vi "WVDIAL_Main.vi"() -> ()   [LabVIEW 2024]
uses:
  TypeDefinitions.llb/TypeDef_MainControlSystem.ctl
  TypeDefinitions.llb/TypeDef_LoopStagesMain.ctl
  <vilib>/Utility/miscctls.llb/LVRectTypeDef.ctl
  <vilib>/Utility/miscctls.llb/LVPointTypeDef.ctl
  TypeDefinitions.llb/TypeDef_ConfigureFIleTypes.ctl
  TypeDefinitions.llb/TypeDef_ChildReporting.ctl
  TypeDefinitions.llb/TypeDef_MainSpecialConfiguration.ctl
  WVDIAL_GlobalVariables.vi
panel:
  out "ChildrenDetails":T2(array[cluster])
  in  "Software Testing":bool
  out "Pages":refnum<vi>[](array[refnum])
  out "SubPanelRefs":refnum<vi>[](array[refnum])
  out "SubPanelWidth":i32=985
  out "SubPanelHeight":i32=540
  out "error IO":errorcluster
  out "Children Responding":T3(array[cluster])
  out "QueueElement":string="Exit"
  out "LoopCounter":i32=200
  out "Permission Level":T4(ring)
  in  "User Comment":bool
  in  "Update Permissions":bool
  in  "Global Abort":bool=TRUE
  in  "Tab Control":T5(tab)
  in  "BDetector":bool=TRUE
  in  "DopFreeScan":bool=TRUE
  out "Doppler Free Calibration":bool
  out "Receiver Calibration":bool
  in  "AfterPulse Calibration":bool
  in  "Aerodiode":bool=TRUE
  in  "TCSPC":bool=TRUE
  in  "CurrentSensor":bool=TRUE
  in  "ConfigThor8000":bool=TRUE caption="ConfigQC"
  in  "ConfigQC":bool=TRUE
  in  "Switches":bool=TRUE
  in  "Wavemeter":bool=TRUE
  in  "Thor8000":bool=TRUE
  in  "PowerSwitches":bool=TRUE
  in  "SetupRScan":bool=TRUE
  in  "Housekeeping":bool=TRUE
  in  "Operations":bool=TRUE
  in  "Warmup":bool=TRUE
  out "DIAL unit":string="DIAL5"
  out "UPSAbort":bool
  in  "NetCDF":bool=TRUE
  in  "Thermocouples":bool=TRUE
  in  "LaserLocking":bool=TRUE
  in  "MCS":bool=TRUE
  in  "Weather Station":bool=TRUE
  in  "QComposer":bool=TRUE
  in  "UPS":bool=TRUE
  in  "Humidity":bool=TRUE
  in  "Template":bool=TRUE
  out "What to Do":string
  out "WritePaths":path[](array[path])=[path "C:/Users/h2odial/Desktop/WVDCode/WVD-MCSupdate/WVDNewArchitectureUpdate/WVD_Architecture_Update/Data/Container/20181008/ContainerLogging_20181008_155204.txt"]
  out "DataBasePath":string="C:\\Users\\h2odial\\Desktop\\WVDCode\\WVD-MCSupdate\\WVDNewArchitectureUpdate\\WVD_Architecture_Update\\Data\\Container\\"
  out "FileBaseNames":string[](array[string])=["ContainerLogging"]
  out "FileUpdateTime":dbl=15.867789441666668
  in  "TempScan":bool=TRUE
  out "First/LastCall":bool
  out "Configuration":enum16{"Ops", "ReceiverScan"}(ring)
  in  "PulsedScan":bool=TRUE
  # "Place Hidden Variables Here"
  # "Main Programs"
  # "Testing Programs"
  # "Hardware Setup Programs"
  # "Individual Controls"
  # "Calibration  Programs"
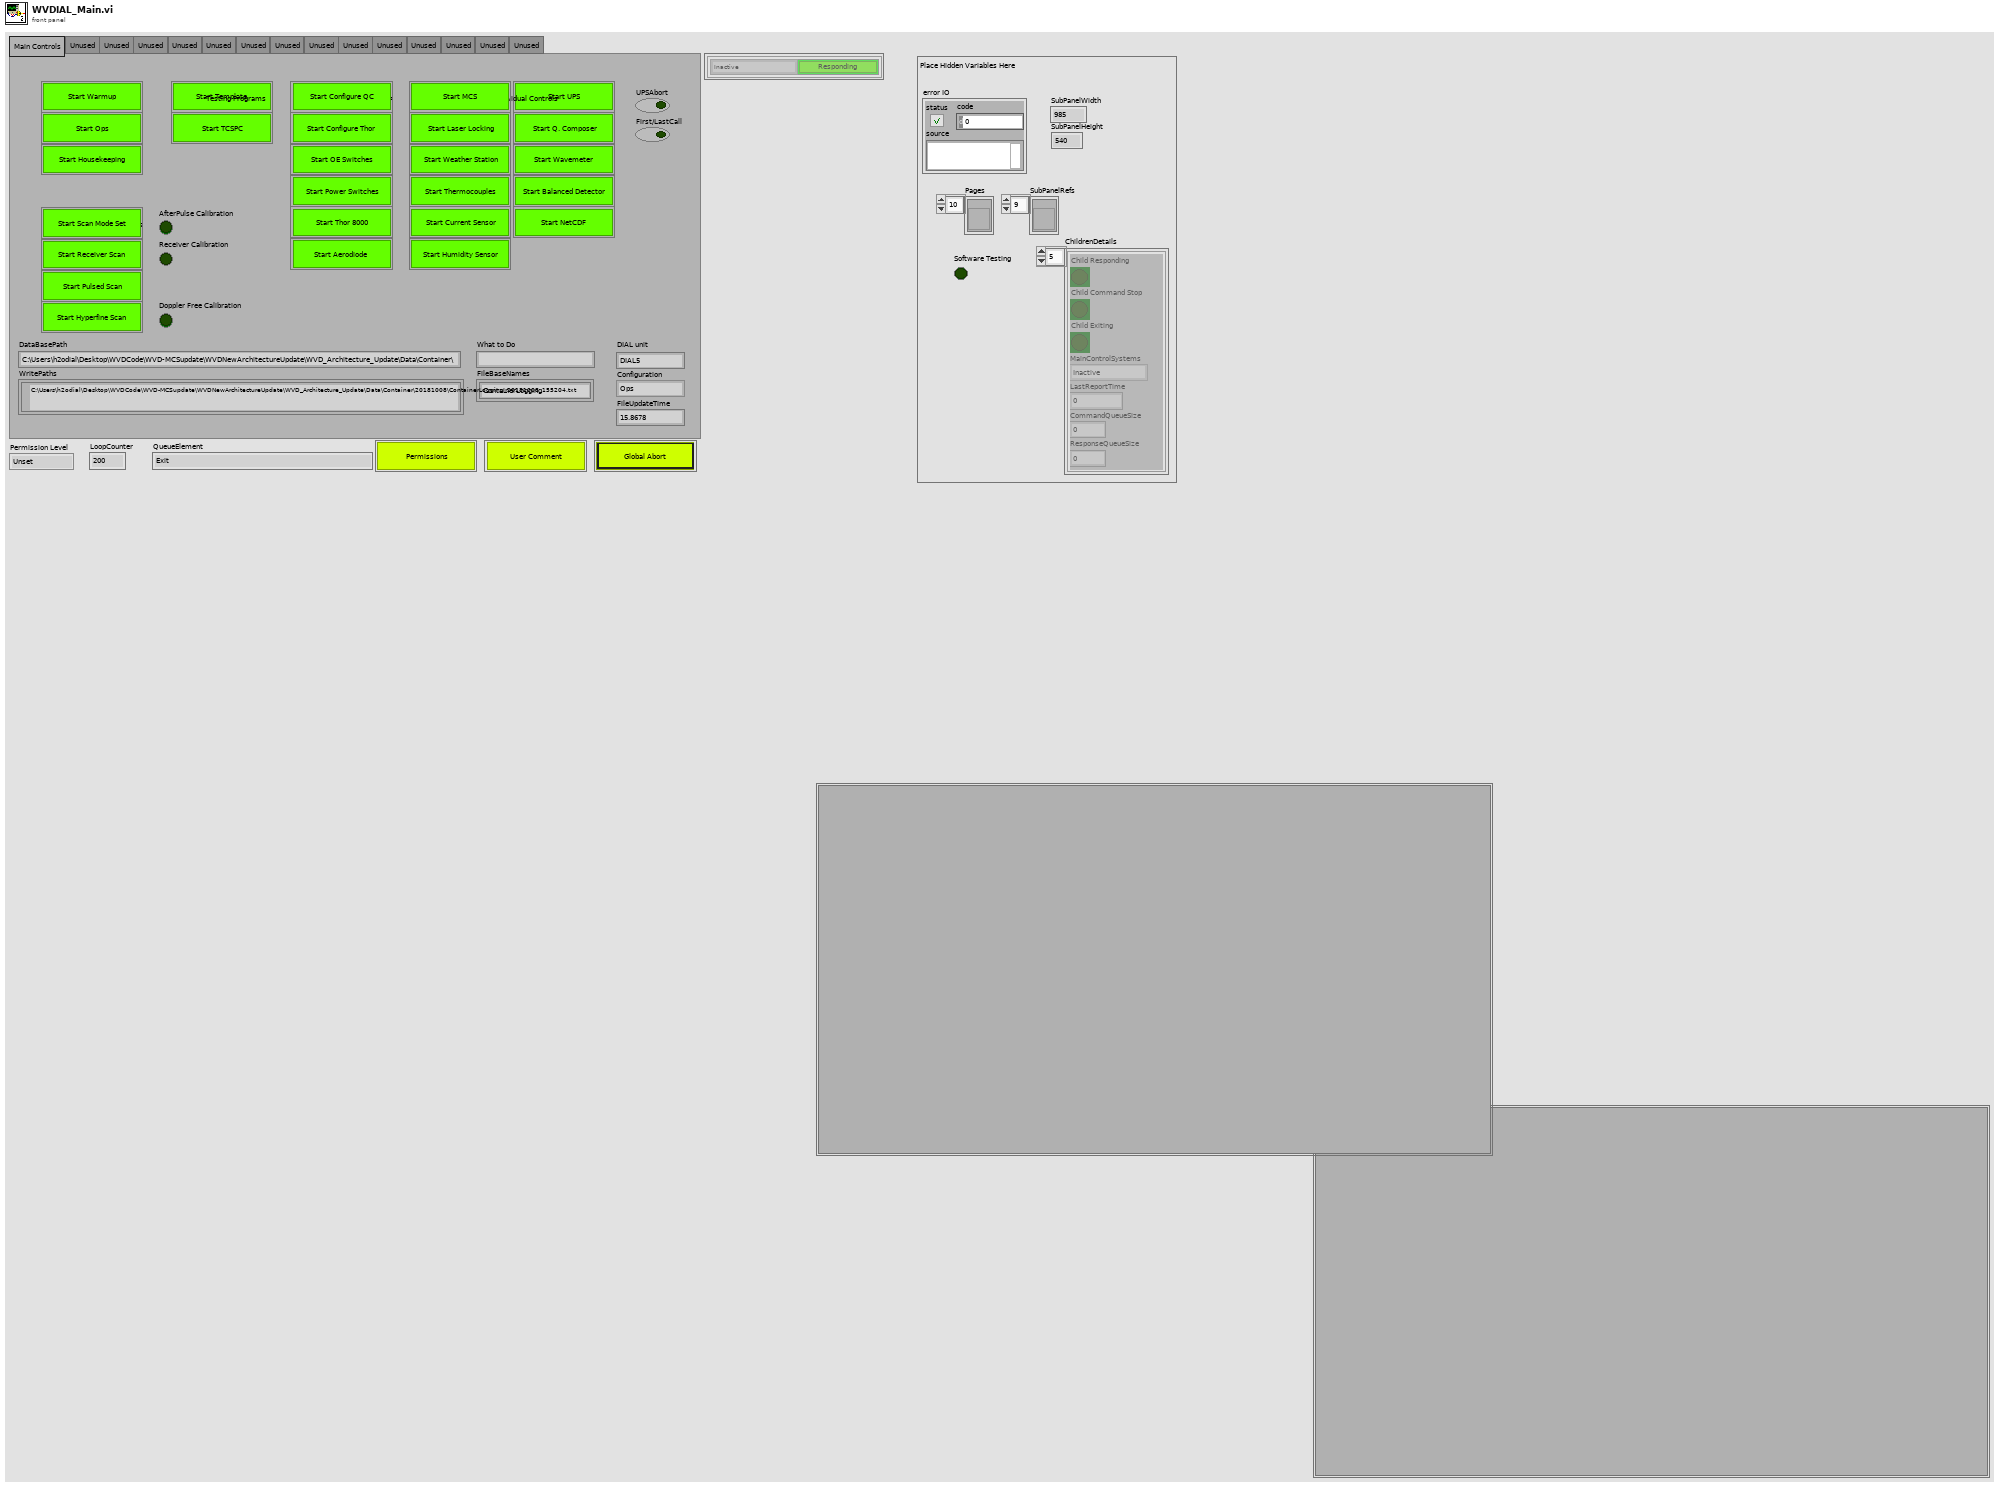
[diagram p1: front panel]
types:
  T1 = typedef "TypeDef_MainControlSystem.ctl" = enum16{"Inactive", "MCS", "MCSControls", "LaserControl", "LaserLocking", "WeatherStation", "DataDisplay", "DataNetCDF", "Template", "WavelengthLocking", "Wavemeter", "Switches", "Thermocouple", "UPS", "PowerSwitches", "Thor8000", "ReceiverScan", "Clock", "HumiditySensor", "SetupReceiverScan", "ConfigureQC", "ConfigureThor8000", "Container", "CurrentSensor", "TCSPC", "Aerodiode", "Balanced Detector", "HVAC"}
  T2 = cluster{"Child Command Stop":bool, "Child Responding":bool, "MainControlSystems":T1, "LastReportTime":dbl, "Child Exiting":bool, "CommandQueueSize":dbl, "ResponseQueueSize":dbl}[]
  T3 = cluster{"MainControlSystems":T1, "Responding":bool}[]
  T4 = enum16{"Unset", "Operator", "Administrator", "Full"}
  T5 = enum32{"Main Controls", "Inner Function 1", "Inner Function 2", "Inner Function 3", "Inner Function 4", "Inner Function 5", "Inner Function 6", "Inner Function 7", "Inner Function 8", "Unused", "Unused 2", "Unused11", "Unused12", "Unused13", "Unused14"}
  T6 = typedef "TypeDef_LoopStagesMain.ctl" = enum16{"Configure", "Initialize", "Set Visibility", "Idle", "ExitChildren", "Error Handler", "Exit"}
  T7 = typedef "TypeDef_ConfigureFIleTypes.ctl" = enum16{"Main", "ConfigureAerodiode", "ConfigureQC", "ConfigureThor8000", "OpsCurrent", "OpsHousekeeping", "OpsHumiditySensor", "OpsHVAC", "OpsMain", "OpsMCS", "OpsNetCDF", "OpsQuantumComposer", "OpsTemplate", "OpsThermocouple", "OpsUPS", "OpsWarmup", "OpsWavlengthLocking", "OpsWeatherStation", "ChildAerodiode", "ChildBalancedDetector", "ChildScanPlotting", "ChildPlotting", "ChildCurrent", "ChildHousekeeping", "ChildHumiditySensor", "ChildHVAC", "ChildLaserLocking", "ChildMCSV2", "ChildNetCDF", "ChildPowerSwitches", "ChildQuantumComposer", "ChildSmartMCS", "ChildSmartSwitch", "ChildSwitches", "ChildTCSPC", "ChildTemplate", "ChildThor8000", "ChildUPS", "ChildWavelengthScanMCS", "ChildWavelengthScanMCX", "ChildWavelengthScanPulsedMCX", "ChildWavelengthScanSmartSwitch", "ChildWavemeter", "ChildWavemeter_Fizeau", "ChildWeatherStation", "TestingBalancedDetector", "TestingHyperFineScan", "TestingPowerSwitches", "TestingReceiverScan", "TestingSetupReceiverScan", "TestingSwitches", "TestingTCSPC", "TestingThor8000", "TestingWavemeter", "EmailList", "SubChildWVPlot", "SubChildWVLowPlot", "SubChildKHSRLPlot", "SubChildO2Plot", "SubChildScanPlot"}
  T8 = typedef "LVPointTypeDef.ctl" = cluster{"Horizontal":i16, "Vertical":i16}
  T9 = typedef "LVRectTypeDef.ctl" = cluster{"Left":i16, "Top":i16, "Right":i16, "Bottom":i16}
  T10 = typedef "TypeDef_ChildReporting.ctl" = cluster{"Child Command Stop":bool, "Child Responding":bool, "MainControlSystems":T1, "LastReportTime":dbl, "Child Exiting":bool, "CommandQueueSize":dbl, "ResponseQueueSize":dbl}
  T11 = enum32{"Page Enabled", "Page Disabled", "Page Disabled & Grayed"}
  T12 = cluster{"MainControlSystems":T1, "Responding":bool}
  T13 = typedef "TypeDef_MainSpecialConfiguration.ctl" = enum16{"Ops", "ReceiverScan", "PulsedScan", "HyperFineScan"}
  T14 = enum16{"Always On", "Always Off", "Off While Running"}
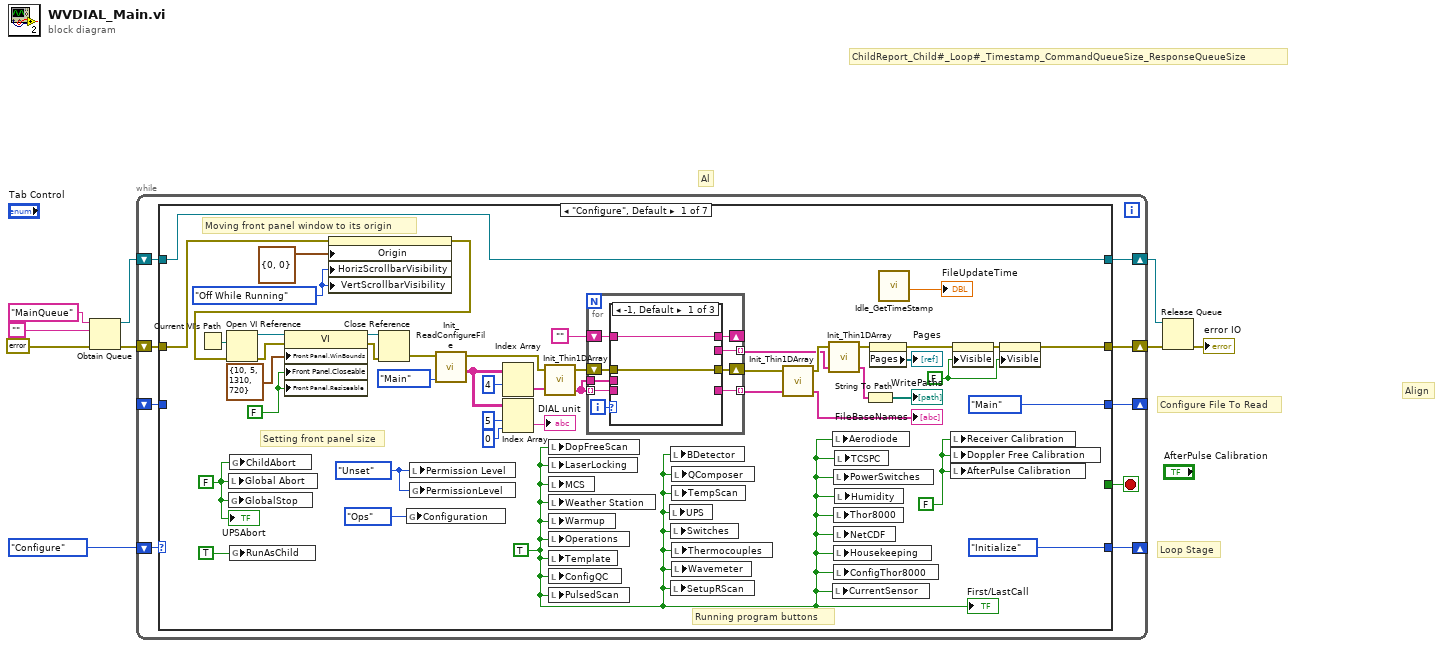
[diagram p0: block diagram]
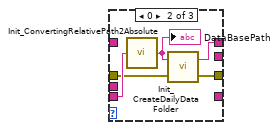
[diagram p2: hidden frame]
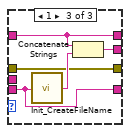
[diagram p3: hidden frame]
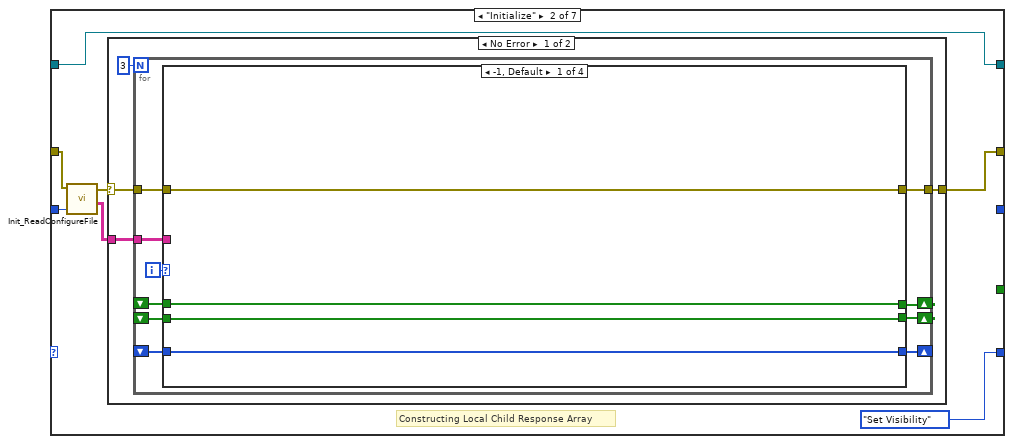
[diagram p4: hidden frame]
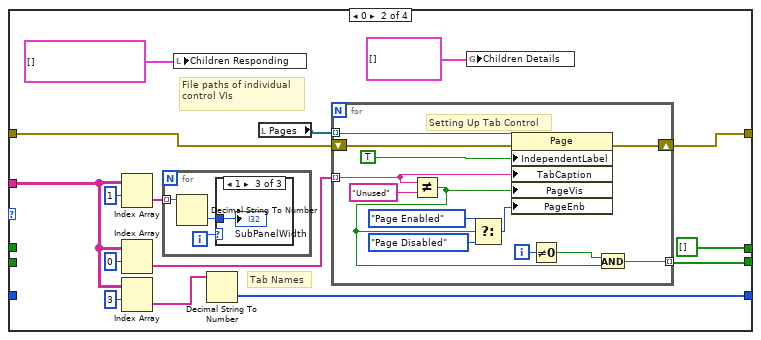
[diagram p5: hidden frame]
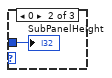
[diagram p7: hidden frame]
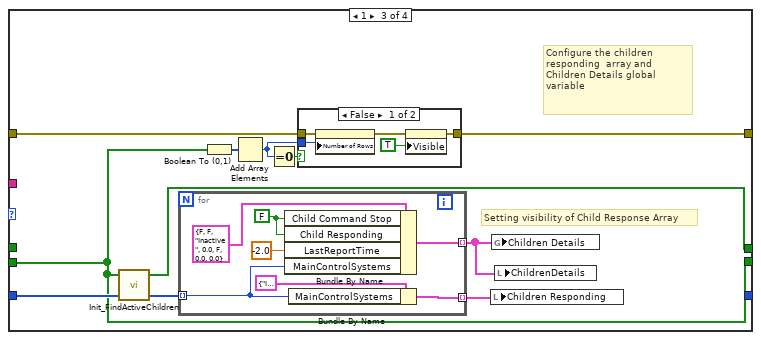
[diagram p8: hidden frame]
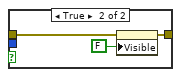
[diagram p9: hidden frame]
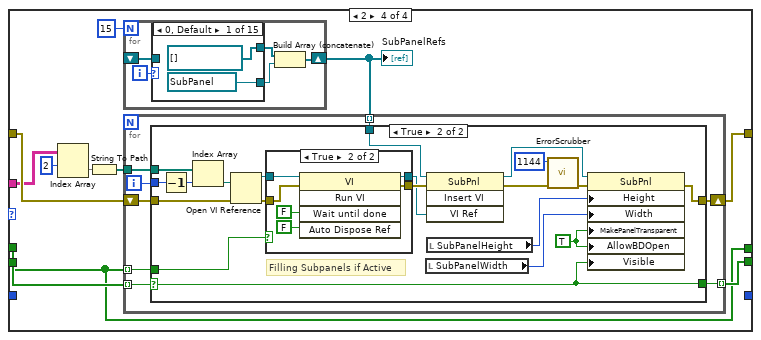
[diagram p10: hidden frame]
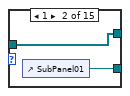
[diagram p11: hidden frame]
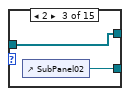
[diagram p12: hidden frame]
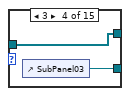
[diagram p13: hidden frame]
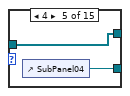
[diagram p14: hidden frame]
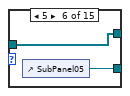
[diagram p15: hidden frame]
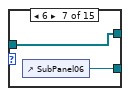
[diagram p16: hidden frame]
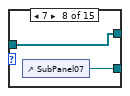
[diagram p17: hidden frame]
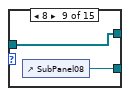
[diagram p18: hidden frame]
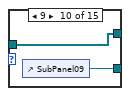
[diagram p19: hidden frame]
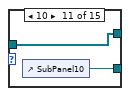
[diagram p20: hidden frame]
diagram:
  # "Al"
  # "Align"
  # "ChildReport_Child#_Loop#_Timestamp_CommandQueueSize_ResponseQueueSize"
  # "Configure File To Read"
  # "Loop Stage"
  n1 = Obtain Queue(name (unnamed)="MainQueue", element data type="", error in (no error)=errorcluster {"status"=FALSE, "code"=0, "source"=""}) -> (queue out=w3:refnum<queue>, error out=w4:errorcluster)  [unwired: 2 in, 1 out]
  n2 = while {
    shift-right: [w14] -> w7
    shift-left: w4 -> [w15]
    shift-right: [w13] -> w8
    shift-left: w3 -> [w12]
    shift-right: [w17] -> _
    shift-left: TypeDef_LoopStagesMain."Configure" ("Enum") -> [w18]
    shift-right: [w11] -> _
    shift-left: _ -> [w10]
    stop <- w16 stop-if-true
    n3 = case shown="\"Configure\", Default" w18 {
      tunnel: [TypeDef_LoopStagesMain."Initialize" ("Enum") TypeDef_LoopStagesMain."Set Visibility" ("Enum") TypeDef_LoopStagesMain."Idle" ("Enum") w462 TypeDef_LoopStagesMain."Initialize" ("Enum") TypeDef_LoopStagesMain."Idle" ("Enum") TypeDef_LoopStagesMain."Exit" ("Enum")] -> w17
      tunnel: [_ _ _ _ _ _ TRUE] -> w16
      tunnel: [w32 w91 w256 w459 w940 w954 w987] -> w14
      tunnel: w15 -> [w51 w90 w257 w463 w939 w953 w981]
      tunnel: [w22 w86 w259 w464 w944 w955 w988] -> w13
      tunnel: w12 -> [w22 w86 w259 w458 w944 w955 w988]
      tunnel: [TypeDef_ConfigureFIleTypes."Main" ("MainControlSystems") _ _ w457 w942 _ _] -> w11
      tunnel: w10 -> [_ w87 _ _ w942 _ _]
      frame "Configure", Default {
        w20 = FALSE
        w31 = FALSE ("Visible")
        w53 = T14."Off While Running" ("Vertical Scrollbar Visibility")
        w60 = FALSE
        w19 = TRUE ("Warmup")
        w61 = T4."Unset" ("Permission Level")
        w34 = FALSE ("Global Stop")
        # "Running program buttons"
        # "Setting front panel size"
        # "Moving front panel window to its origin"
        n4 = Current VI's Path() -> (path=w54:path)
        n5 = local write "Global Abort"(w34) -> ()
        n6 = global write "WVDIAL_GlobalVariables.vi" "GlobalStop"(w34) -> ()
        n7 = global write "WVDIAL_GlobalVariables.vi" "ChildAbort"(w34) -> ()
        n8 = global write "WVDIAL_GlobalVariables.vi" "RunAsChild"(TRUE ("RunAsChild")) -> ()
        n9 = property on="Pane" class="Pane"(error in=w51, "Origin"=T8 {"Horizontal"=0, "Vertical"=0}, "HorizScrollbarVisibility"=w53, "VertScrollbarVisibility"=w53) -> (error out=w23:errorcluster)  [unwired: 1 in, 1 out]
        n10 = Open VI Reference(vi path=w54, error in (no error)=w23) -> (vi reference=w55:refnum<vi>, error out=w56:errorcluster)  [unwired: 4 in]
        n11 = property class="VI"(reference=w55, error in=w56, "Front Panel.WinBounds"=T9 {"Left"=10, "Top"=5, "Right"=1310, "Bottom"=720} ("Front Panel Window:Panel Bounds"), "Front Panel.Closeable"=w60, "Front Panel.Resizeable"=w60) -> (reference out=w57:refnum<vi>, error out=w58:errorcluster)
        n12 = Close Reference(reference=w57, error in (no error)=w58) -> (error out=w47:errorcluster)
        n13 = global write "WVDIAL_GlobalVariables.vi" "Configuration"(enum16{"Ops", "ReceiverScan"}."Ops" ("Configuration")) -> ()
        n14 = local write "Permission Level"(w61) -> ()
        n15 = global write "WVDIAL_GlobalVariables.vi" "PermissionLevel"(w61) -> ()
        n16 = call "Init_ReadConfigureFile.vi"("ConfigureFileType"=TypeDef_ConfigureFIleTypes."Main" ("MainControlSystems"), "ErrorIn"=w47) -> ("Parsed List"=w27:string[][], "ErrorOut"=w25:errorcluster)  [unwired: 4 in, 2 out]
        n17 = Index Array(array=w27, index (row)=4) -> (element=w48:string[])  [unwired: 1 in]
        n18 = Index Array(array=w27, index (row)=5, index (col)=0 ("disabled index (col)")) -> (element=→"DIAL unit":string)
        n19 = call "Init_Thin1DArray.vi"("Padded Array"=w48, "ErrorIn"=w25) -> ("ThinnedArray"=w43:string[], "ErrorOut"=w45:errorcluster)  [unwired: 1 in, 1 out]
        n20 = local write "DopFreeScan"(w19) -> ()
        n21 = local write "LaserLocking"(w19) -> ()
        n22 = local write "MCS"(w19) -> ()
        n23 = local write "Weather Station"(w19) -> ()
        n24 = local write "Warmup"(w19) -> ()
        n25 = local write "Operations"(w19) -> ()
        n26 = local write "Template"(w19) -> ()
        n27 = local write "ConfigQC"(w19) -> ()
        n28 = local write "PulsedScan"(w19) -> ()
        n29 = for {
          shift-right: [w70] -> w26
          shift-left: w45 -> [w71]
          tunnel: w43 -> [w72] mode=indexing
          shift-right: [w69] -> _
          shift-left: "" -> [w68]
          tunnel: [w67] -> w38 mode=indexing
          tunnel: [w66] -> w39 mode=indexing
          tunnel: w43 -> [w65]
          i -> [w73]
          n30 = case shown="-1, Default" w73 {
            tunnel: w72 -> [_ w80 w82]
            tunnel: w71 -> [w74 w78 w84]
            tunnel: [w74 w77 w84] -> w70
            tunnel: [w75 w79 w83] -> w69
            tunnel: w68 -> [w75 _ w83]
            tunnel: [_ _ w82] -> w67
            tunnel: [_ _ w81] -> w66
            tunnel: w65 -> [_ _ _]
            frame -1, Default {
            }
            frame 0 {
              n31 = call "Init_ConvertingRelativePath2Absolute.vi"("PathFromConfigureFileIn"=w80) -> ("PathOut"=w76:string)
              "DataBasePath" <- w76
              n32 = call "Init_CreateDailyDataFolder.vi"("ErrorIn"=w78, "PathIn"=w76) -> ("ErrorOut"=w77:errorcluster, "PathOut"=w79:string)
            }
            frame 1 {
              n33 = call "Init_CreateFileName.vi"("BaseFileName"=w82) -> ("FileName"=w85:string)
              n34 = Concatenate Strings(w83, w85) -> (w81:string)
            }
          }
        }
        n35 = local write "UPS"(w19) -> ()
        n36 = local write "BDetector"(w19) -> ()
        n37 = local write "Switches"(w19) -> ()
        n38 = local write "SetupRScan"(w19) -> ()
        n39 = local write "QComposer"(w19) -> ()
        n40 = local write "TempScan"(w19) -> ()
        n41 = local write "Thermocouples"(w19) -> ()
        n42 = local write "Wavemeter"(w19) -> ()
        n43 = call "Init_Thin1DArray.vi"("Padded Array"=w38, "ErrorIn"=w26) -> ("ThinnedArray"=→"FileBaseNames":string[], "ErrorOut"=w40:errorcluster)  [unwired: 1 in, 1 out]
        n44 = call "Init_Thin1DArray.vi"("Padded Array"=w39, "ErrorIn"=w40) -> ("ThinnedArray"=w41:string[], "ErrorOut"=w36:errorcluster)  [unwired: 1 in, 1 out]
        n45 = local write "Aerodiode"(w19) -> ()
        n46 = local write "CurrentSensor"(w19) -> ()
        n47 = local write "PowerSwitches"(w19) -> ()
        n48 = local write "Thor8000"(w19) -> ()
        n49 = local write "NetCDF"(w19) -> ()
        n50 = local write "Housekeeping"(w19) -> ()
        n51 = local write "ConfigThor8000"(w19) -> ()
        n52 = local write "TCSPC"(w19) -> ()
        n53 = local write "Humidity"(w19) -> ()
        n54 = String To Path(string=w41) -> (path=→"WritePaths":path[])
        n55 = property on="Tab Control" class="TabCtl (strict)"(error in=w36) -> (error out=w24:errorcluster, "Pages"=→"Pages":refnum<vi>[])  [unwired: 1 in, 1 out]
        n56 = call "Idle_GetTimeStamp.vi"() -> ("Fractional Hours"=→"FileUpdateTime":dbl)  [unwired: 11 in]
        n57 = local write "Receiver Calibration"(w20) -> ()
        n58 = local write "Doppler Free Calibration"(w20) -> ()
        n59 = local write "AfterPulse Calibration"(w20) -> ()
        n60 = property on="First/LastCall" class="Bool (strict)"(error in=w24, "Visible"=w31) -> (error out=w33:errorcluster)  [unwired: 1 in, 1 out]
        n61 = property on="UPSAbort" class="Bool (strict)"(error in=w33, "Visible"=w31) -> (error out=w32:errorcluster)  [unwired: 1 in, 1 out]
        "First/LastCall" <- w19
        "UPSAbort" <- w34
      }
      frame "Initialize" {
        # "Constructing Local Child Response Array"
        n62 = call "Init_ReadConfigureFile.vi"("ConfigureFileType"=w87, "ErrorIn"=w90) -> ("Parsed List"=w88:string[][], "ErrorOut"=w89:errorcluster)  [unwired: 4 in, 2 out]
        n63 = case shown="No Error" w89 {
          selector: w89 -> [w95 w254]
          tunnel: [w96 w254] -> w91
          tunnel: w88 -> [w94 _]
          frame No Error {
            n64 = for {
              N: 3 -> [_]
              tunnel: [w106] -> w96
              tunnel: w95 -> [w101]
              tunnel: w94 -> [w104]
              shift-right: [w103] -> _
              shift-left: _ -> [w102]
              shift-right: [w100] -> _
              shift-left: _ -> [w99]
              shift-right: [w98] -> _
              shift-left: _ -> [w97]
              i -> [w105]
              n65 = case shown="-1, Default" w105 {
                tunnel: [w110 w111 w151 w180] -> w106
                tunnel: w101 -> [w110 w115 w152 w178]
                tunnel: w104 -> [_ w112 _ w170]
                tunnel: [w109 w121 w147 w177] -> w103
                tunnel: w102 -> [w109 _ w147 w179]
                tunnel: [w108 w118 _ _] -> w100
                tunnel: w99 -> [w108 _ w148 _]
                tunnel: [w107 bool[] [] ("StartSubVI") w145 w174] -> w98
                tunnel: w97 -> [w107 _ _ w174]
                frame -1, Default {
                }
                frame 0 {
                  # "File paths of individual control VIs"
                  # "Tab Names"
                  n66 = Index Array(array=w112, index (row)=1) -> (element=w123:string[])  [unwired: 1 in]
                  n67 = Index Array(array=w112, index (row)=0) -> (element=w122:string[])  [unwired: 1 in]
                  n68 = Index Array(array=w112, index (row)=3) -> (element=w119:string[])  [unwired: 1 in]
                  n69 = for {
                    tunnel: w123 -> [w140] mode=indexing
                    i -> [w141]
                    n70 = Decimal String To Number(string=w140) -> (number=w139:i32)  [unwired: 2 in, 1 out]
                    n71 = case shown="1" w141 {
                      tunnel: w139 -> [_ w142 w143]
                      frame -1, Default {
                      }
                      frame 0 {
                        "SubPanelHeight" <- w142
                      }
                      frame 1 {
                        "SubPanelWidth" <- w143
                      }
                    }
                  }
                  n72 = local write "Children Responding"(T3 [] ("Children Responding")) -> ()
                  n73 = Decimal String To Number(string=w119) -> (number=w118:i32[])  [unwired: 2 in, 1 out]
                  n74 = local read "Pages"() -> (w116:refnum<vi>[])
                  n75 = for {
                    tunnel: w122 -> [w132] mode=indexing
                    tunnel: w116 -> [w135] mode=indexing
                    shift-right: [w133] -> w111
                    shift-left: w115 -> [w134]
                    tunnel: [w129] -> w121 mode=indexing
                    i -> [w130]
                    # "Setting Up Tab Control"
                    n76 = Not Equal?(x=w132, y="Unused") -> (x != y?=w127:bool)
                    n77 = Select(t=T11."Page Enabled" ("Page Enabled State"), s=w127, f=T11."Page Disabled" ("Page Enabled State")) -> (s? t:f=w126:T11)
                    n78 = property class="Page"(reference=w135, error in=w134, "IndependentLabel"=TRUE ("Independent Label"), "TabCaption"=w132, "PageVis"=w127, "PageEnb"=w126) -> (error out=w133:errorcluster)  [unwired: 1 out]
                    n79 = Not Equal To 0?(x=w130) -> (x != 0?=w131:bool)
                    n80 = And(x=w131, y=w127) -> (x .and. y?=w129:bool)
                  }
                  n81 = global write "WVDIAL_GlobalVariables.vi" "Children Details"(T10[] [] ("Children Details")) -> ()
                }
                frame 1 {
                  # "Setting visibility of Child Response Array"
                  # "Configure the children responding  array and Children Details global variable"
                  n82 = call "Init_FindActiveChildren.vi"("ChannelType"=w148, "ChannelOn"=w147) -> ("ActiveTypes"=w146:i32[], "StartSubVI"=w145:bool[])  [unwired: 1 in, 1 out]
                  n83 = for {
                    tunnel: [w168] -> w153 mode=indexing
                    tunnel: w146 -> [w164] mode=indexing
                    tunnel: [w167] -> w144 mode=indexing
                    w166 = FALSE
                    n84 = Bundle By Name(cluster=T10 {"Child Command Stop"=FALSE, "Child Responding"=FALSE, "MainControlSystems"=enum."Inactive", "LastReportTime"=0.0, "Child Exiting"=FALSE, "CommandQueueSize"=0.0, "ResponseQueueSize"=0.0} ("Child Details"), "Child Command Stop"=w166, "Child Responding"=w166, "LastReportTime"=-2.0, "MainControlSystems"=w164) -> (w167:T10)
                    n85 = Bundle By Name(cluster=T12 {"MainControlSystems"=enum."Inactive", "Responding"=TRUE} ("ChildResponse"), "MainControlSystems"=w164) -> (w168:T12)
                  }
                  n86 = Boolean To (0,1)(Boolean=w147) -> (0, 1=w154:i16[])
                  n87 = Add Array Elements(numeric array=w154) -> (sum=w150:i16)
                  n88 = Equal To 0?(x=w150) -> (x = 0?=w149:bool)
                  n89 = case shown="False" w149 {
                    tunnel: w152 -> [w159 w162]
                    tunnel: [w156 w161] -> w151
                    tunnel: w150 -> [w158 _]
                    frame False {
                      n90 = property on="Children Responding" class="Arr (strict)"(error in=w159, "Number of Rows"=w158) -> (error out=w157:errorcluster)  [unwired: 1 in, 1 out]
                      n91 = property on="Children Responding" class="Arr (strict)"(error in=w157, "Visible"=TRUE) -> (error out=w156:errorcluster)  [unwired: 1 in, 1 out]
                    }
                    frame True {
                      n92 = property on="Children Responding" class="Arr (strict)"(error in=w162, "Visible"=FALSE) -> (error out=w161:errorcluster)  [unwired: 1 in, 1 out]
                    }
                  }
                  n93 = local write "Children Responding"(w153) -> ()
                  n94 = global write "WVDIAL_GlobalVariables.vi" "Children Details"(w144) -> ()
                  n95 = local write "ChildrenDetails"(w144) -> ()
                }
                frame 2 {
                  n96 = Index Array(array=w170, index (row)=2) -> (element=w173:string[])  [unwired: 1 in]
                  n97 = String To Path(string=w173) -> (path=w171:path[])
                  n98 = for {
                    N: 15 -> [_]
                    shift-right: [w185] -> w175
                    shift-left: _ -> [w181]
                    i -> [w184]
                    n99 = case shown="0, Default" w184 {
                      tunnel: [refnum<vi> refnum ("SubPanel8") w189 w191 w193 w195 w197 w199 w201 w203 w205 w207 w208 w210 w212 w214] -> w183
                      tunnel: [refnum<vi>[] [] w188 w190 w192 w194 w196 w198 w200 w202 w204 w206 w209 w211 w213 w215] -> w182
                      tunnel: w181 -> [_ w188 w190 w192 w194 w196 w198 w200 w202 w204 w206 w209 w211 w213 w215]
                      frame 0, Default {
                      }
                      frame 1 {
                        n100 = control-ref of="SubPanel01"() -> (w189:refnum<vi>)
                      }
                      frame 2 {
                        n101 = control-ref of="SubPanel02"() -> (w191:refnum<vi>)
                      }
                      frame 3 {
                        n102 = control-ref of="SubPanel03"() -> (w193:refnum<vi>)
                      }
                      frame 4 {
                        n103 = control-ref of="SubPanel04"() -> (w195:refnum<vi>)
                      }
                      frame 5 {
                        n104 = control-ref of="SubPanel05"() -> (w197:refnum<vi>)
                      }
                      frame 6 {
                        n105 = control-ref of="SubPanel06"() -> (w199:refnum<vi>)
                      }
                      frame 7 {
                        n106 = control-ref of="SubPanel07"() -> (w201:refnum<vi>)
                      }
                      frame 8 {
                        n107 = control-ref of="SubPanel08"() -> (w203:refnum<vi>)
                      }
                      frame 9 {
                        n108 = control-ref of="SubPanel09"() -> (w205:refnum<vi>)
                      }
                      frame 10 {
                        n109 = control-ref of="SubPanel10"() -> (w207:refnum<vi>)
                      }
                      frame 11 {
                        n110 = control-ref of="SubPanel11"() -> (w208:refnum<vi>)
                      }
                      frame 12 {
                        n111 = control-ref of="SubPanel12"() -> (w210:refnum<vi>)
                      }
                      frame 13 {
                        n112 = control-ref of="SubPanel13"() -> (w212:refnum<vi>)
                      }
                      frame 14 {
                        n113 = control-ref of="SubPanel14"() -> (w214:refnum<vi>)
                      }
                    }
                    n114 = Build Array (concatenate)(w182, w183) -> (w185:refnum<vi>[])
                  }
                  "SubPanelRefs" <- w175
                  n115 = for {
                    shift-right: [w222] -> w180
                    shift-left: w178 -> [w223]
                    tunnel: w171 -> [w221]
                    tunnel: w179 -> [w218] mode=indexing
                    tunnel: [w220] -> w177 mode=indexing
                    tunnel: w175 -> [w217] mode=indexing
                    tunnel: w174 -> [w216] mode=indexing
                    i -> [w219]
                    n116 = case shown="True" w218 {
                      selector: w218 -> [w224 w231]
                      tunnel: w223 -> [w225 w245]
                      tunnel: [w225 w233] -> w222
                      tunnel: w221 -> [_ w244]
                      tunnel: w219 -> [_ w236]
                      tunnel: [w224 w231] -> w220
                      tunnel: w217 -> [_ w234]
                      tunnel: w216 -> [_ w230]
                      frame False {
                      }
                      frame True {
                        w237 = TRUE ("Allow User to Open Diagram")
                        # "Filling Subpanels if Active"
                        n117 = Decrement(x=w236) -> (x-1=w235:i32)
                        n118 = Index Array(array=w244, index=w235) -> (element=w243:path)
                        n119 = Open VI Reference(vi path=w243, error in (no error)=w245) -> (vi reference=w242:refnum<vi>, error out=w241:errorcluster)  [unwired: 4 in]
                        n120 = case shown="True" w230 {
                          tunnel: w242 -> [w247 w253]
                          tunnel: w241 -> [w246 w252]
                          tunnel: [w246 w250] -> w240
                          tunnel: [w247 w248] -> w232
                          frame False {
                          }
                          frame True {
                            n121 = invoke class="VI" method="Run VI"(reference=w253, error in=w252, "Wait until done"=FALSE ("Wait Until Done"), "Auto Dispose Ref"=FALSE ("Auto Dispose Reference")) -> (reference out=w248:refnum<vi>, error out=w250:errorcluster)  [unwired: 1 in, 3 out]
                          }
                        }
                        n122 = local read "SubPanelWidth"() -> (w238:i32)
                        n123 = invoke on="Invoke Node" class="SubPnl" method="Insert VI"(reference=w234, error in=w240, "VI Ref"=w232) -> (reference out=w226:refnum<vi>, error out=w228:errorcluster)  [unwired: 1 in, 2 out]
                        n124 = local read "SubPanelHeight"() -> (w239:i32)
                        n125 = call "ErrorScrubber.vi"("error in (no error)"=w228, "y"=1144) -> ("error out"=w229:errorcluster)  [unwired: 8 in, 1 out]
                        n126 = property on="Property Node" class="SubPnl"(reference=w226, error in=w229, "Height"=w239, "Width"=w238, "MakePanelTransparent"=w237, "AllowBDOpen"=w237, "Visible"=w231) -> (error out=w233:errorcluster)  [unwired: 1 out]
                      }
                    }
                  }
                }
              }
            }
          }
          frame Error {
          }
        }
      }
      frame "Set Visibility" {
        # "Al"
        # "Al"
        n127 = local read "First/LastCall"() -> (w255:bool)
        n128 = case shown="False" w255 {
          selector: w255 -> [w260 w373]
          tunnel: w257 -> [w263 w376]
          tunnel: [w262 w375] -> w256
          frame False {
            n129 = for {
              N: 26 -> [_]
              shift-right: [w266] -> w262
              shift-left: w263 -> [w265]
              i -> [w267]
              n130 = case shown="25" w267 {
                tunnel: [w268 w272 w276 w278 w283 w287 w291 w293 w299 w303 w307 w311 w313 w317 w321 w325 w329 w333 w339 w343 w346 w350 w354 w357 w361 w365 w369] -> w266
                tunnel: w265 -> [w268 w271 w275 w279 w282 w286 w290 w295 w298 w302 w306 w310 w315 w318 w322 w327 w330 w334 w338 w342 w345 w351 w353 w358 w362 w366 w370]
                frame -1, Default {
                }
                frame 0 {
                  n131 = local read "Template"() -> (w269:bool)
                  n132 = Not(x=w269) -> (.not. x?=w270:bool)
                  n133 = property on="Template" class="Bool (strict)"(error in=w271, "Visible"=w270) -> (error out=w272:errorcluster)  [unwired: 1 in, 1 out]
                }
                frame 1 {
                  n134 = local read "Warmup"() -> (w274:bool)
                  n135 = Not(x=w274) -> (.not. x?=w273:bool)
                  n136 = property on="Warmup" class="Bool (strict)"(error in=w275, "Visible"=w273) -> (error out=w276:errorcluster)  [unwired: 1 in, 1 out]
                }
                frame 2 {
                  n137 = local read "Operations"() -> (w280:bool)
                  n138 = Not(x=w280) -> (.not. x?=w277:bool)
                  n139 = property on="Operations" class="Bool (strict)"(error in=w279, "Visible"=w277) -> (error out=w278:errorcluster)  [unwired: 1 in, 1 out]
                }
                frame 3 {
                  n140 = local read "Weather Station"() -> (w284:bool)
                  n141 = Not(x=w284) -> (.not. x?=w281:bool)
                  n142 = property on="Weather Station" class="Bool (strict)"(error in=w282, "Visible"=w281) -> (error out=w283:errorcluster)  [unwired: 1 in, 1 out]
                }
                frame 4 {
                  n143 = local read "MCS"() -> (w288:bool)
                  n144 = Not(x=w288) -> (.not. x?=w285:bool)
                  n145 = property on="MCS" class="Bool (strict)"(error in=w286, "Visible"=w285) -> (error out=w287:errorcluster)  [unwired: 1 in, 1 out]
                }
                frame 5 {
                  n146 = local read "LaserLocking"() -> (w292:bool)
                  n147 = Not(x=w292) -> (.not. x?=w289:bool)
                  n148 = property on="LaserLocking" class="Bool (strict)"(error in=w290, "Visible"=w289) -> (error out=w291:errorcluster)  [unwired: 1 in, 1 out]
                }
                frame 6 {
                  n149 = local read "Wavemeter"() -> (w296:bool)
                  n150 = Not(x=w296) -> (.not. x?=w294:bool)
                  n151 = property on="Wavemeter" class="Bool (strict)"(error in=w295, "Visible"=w294) -> (error out=w293:errorcluster)  [unwired: 1 in, 1 out]
                }
                frame 7 {
                  n152 = local read "Thermocouples"() -> (w300:bool)
                  n153 = Not(x=w300) -> (.not. x?=w297:bool)
                  n154 = property on="Thermocouples" class="Bool (strict)"(error in=w298, "Visible"=w297) -> (error out=w299:errorcluster)  [unwired: 1 in, 1 out]
                }
                frame 8 {
                  n155 = local read "Switches"() -> (w304:bool)
                  n156 = Not(x=w304) -> (.not. x?=w301:bool)
                  n157 = property on="Switches" class="Bool (strict)"(error in=w302, "Visible"=w301) -> (error out=w303:errorcluster)  [unwired: 1 in, 1 out]
                }
                frame 9 {
                  n158 = local read "QComposer"() -> (w308:bool)
                  n159 = Not(x=w308) -> (.not. x?=w305:bool)
                  n160 = property on="QComposer" class="Bool (strict)"(error in=w306, "Visible"=w305) -> (error out=w307:errorcluster)  [unwired: 1 in, 1 out]
                }
                frame 10 {
                  n161 = local read "UPS"() -> (w312:bool)
                  n162 = Not(x=w312) -> (.not. x?=w309:bool)
                  n163 = property on="UPS" class="Bool (strict)"(error in=w310, "Visible"=w309) -> (error out=w311:errorcluster)  [unwired: 1 in, 1 out]
                }
                frame 11 {
                  n164 = local read "PowerSwitches"() -> (w316:bool)
                  n165 = Not(x=w316) -> (.not. x?=w314:bool)
                  n166 = property on="PowerSwitches" class="Bool (strict)"(error in=w315, "Visible"=w314) -> (error out=w313:errorcluster)  [unwired: 1 in, 1 out]
                }
                frame 12 {
                  n167 = local read "Thor8000"() -> (w320:bool)
                  n168 = Not(x=w320) -> (.not. x?=w319:bool)
                  n169 = property on="Thor8000" class="Bool (strict)"(error in=w318, "Visible"=w319) -> (error out=w317:errorcluster)  [unwired: 1 in, 1 out]
                }
                frame 13 {
                  n170 = local read "Humidity"() -> (w324:bool)
                  n171 = Not(x=w324) -> (.not. x?=w323:bool)
                  n172 = property on="Humidity" class="Bool (strict)"(error in=w322, "Visible"=w323) -> (error out=w321:errorcluster)  [unwired: 1 in, 1 out]
                }
                frame 14 {
                  n173 = local read "TempScan"() -> (w328:bool)
                  n174 = Not(x=w328) -> (.not. x?=w326:bool)
                  n175 = property on="TempScan" class="Bool (strict)"(error in=w327, "Visible"=w326) -> (error out=w325:errorcluster)  [unwired: 1 in, 1 out]
                }
                frame 15 {
                  n176 = local read "NetCDF"() -> (w332:bool)
                  n177 = Not(x=w332) -> (.not. x?=w331:bool)
                  n178 = property on="NetCDF" class="Bool (strict)"(error in=w330, "Visible"=w331) -> (error out=w329:errorcluster)  [unwired: 1 in, 1 out]
                }
                frame 16 {
                  n179 = local read "Housekeeping"() -> (w336:bool)
                  n180 = Not(x=w336) -> (.not. x?=w335:bool)
                  n181 = property on="Housekeeping" class="Bool (strict)"(error in=w334, "Visible"=w335) -> (error out=w333:errorcluster)  [unwired: 1 in, 1 out]
                }
                frame 17 {
                  n182 = local read "SetupRScan"() -> (w340:bool)
                  n183 = Not(x=w340) -> (.not. x?=w337:bool)
                  n184 = property on="SetupRScan" class="Bool (strict)"(error in=w338, "Visible"=w337) -> (error out=w339:errorcluster)  [unwired: 1 in, 1 out]
                }
                frame 18 {
                  n185 = local read "ConfigQC"() -> (w344:bool)
                  n186 = Not(x=w344) -> (.not. x?=w341:bool)
                  n187 = property on="ConfigQC" class="Bool (strict)"(error in=w342, "Visible"=w341) -> (error out=w343:errorcluster)  [unwired: 1 in, 1 out]
                }
                frame 19 {
                  n188 = local read "ConfigThor8000"() -> (w348:bool)
                  n189 = Not(x=w348) -> (.not. x?=w347:bool)
                  n190 = property on="ConfigThor8000" class="Bool (strict)"(error in=w345, "Visible"=w347) -> (error out=w346:errorcluster)  [unwired: 1 in, 1 out]
                }
                frame 20 {
                  n191 = local read "CurrentSensor"() -> (w352:bool)
                  n192 = Not(x=w352) -> (.not. x?=w349:bool)
                  n193 = property on="CurrentSensor" class="Bool (strict)"(error in=w351, "Visible"=w349) -> (error out=w350:errorcluster)  [unwired: 1 in, 1 out]
                }
                frame 21 {
                  n194 = local read "TCSPC"() -> (w356:bool)
                  n195 = Not(x=w356) -> (.not. x?=w355:bool)
                  n196 = property on="TCSPC" class="Bool (strict)"(error in=w353, "Visible"=w355) -> (error out=w354:errorcluster)  [unwired: 1 in, 1 out]
                }
                frame 22 {
                  n197 = local read "Aerodiode"() -> (w360:bool)
                  n198 = Not(x=w360) -> (.not. x?=w359:bool)
                  n199 = property on="Aerodiode" class="Bool (strict)"(error in=w358, "Visible"=w359) -> (error out=w357:errorcluster)  [unwired: 1 in, 1 out]
                }
                frame 23 {
                  n200 = local read "BDetector"() -> (w364:bool)
                  n201 = Not(x=w364) -> (.not. x?=w363:bool)
                  n202 = property on="BDetector" class="Bool (strict)"(error in=w362, "Visible"=w363) -> (error out=w361:errorcluster)  [unwired: 1 in, 1 out]
                }
                frame 24 {
                  n203 = local read "DopFreeScan"() -> (w368:bool)
                  n204 = Not(x=w368) -> (.not. x?=w367:bool)
                  n205 = property on="DopFreeScan" class="Bool (strict)"(error in=w366, "Visible"=w367) -> (error out=w365:errorcluster)  [unwired: 1 in, 1 out]
                }
                frame 25 {
                  n206 = local read "PulsedScan"() -> (w372:bool)
                  n207 = Not(x=w372) -> (.not. x?=w371:bool)
                  n208 = property on="PulsedScan" class="Bool (strict)"(error in=w370, "Visible"=w371) -> (error out=w369:errorcluster)  [unwired: 1 in, 1 out]
                }
              }
            }
            n209 = Not(x=w260) -> (.not. x?=w261:bool)
            n210 = local write "First/LastCall"(w261) -> ()
          }
          frame True {
            n211 = for {
              N: 25 -> [_]
              shift-right: [w379] -> w375
              shift-left: w376 -> [w378]
              i -> [w380]
              n212 = case shown="24" w380 {
                tunnel: [w381 w384 w387 w389 w393 w396 w399 w401 w405 w408 w411 w414 w416 w419 w422 w425 w428 w431 w434 w436 w439 w442 w445 w450 w452 w456] -> w379
                tunnel: w378 -> [w381 w383 w386 w390 w392 w395 w398 w402 w404 w407 w410 w413 w417 w420 w423 w426 w429 w432 w433 w437 w440 w443 w446 w448 w451 w455]
                frame -1, Default {
                }
                frame 0 {
                  n213 = local read "Template"() -> (w382:bool)
                  n214 = property on="Template" class="Bool (strict)"(error in=w383, "Visible"=w382) -> (error out=w384:errorcluster)  [unwired: 1 in, 1 out]
                }
                frame 1 {
                  n215 = local read "Warmup"() -> (w385:bool)
                  n216 = property on="Warmup" class="Bool (strict)"(error in=w386, "Visible"=w385) -> (error out=w387:errorcluster)  [unwired: 1 in, 1 out]
                }
                frame 2 {
                  n217 = local read "Operations"() -> (w388:bool)
                  n218 = property on="Operations" class="Bool (strict)"(error in=w390, "Visible"=w388) -> (error out=w389:errorcluster)  [unwired: 1 in, 1 out]
                }
                frame 3 {
                  n219 = local read "Weather Station"() -> (w391:bool)
                  n220 = property on="Weather Station" class="Bool (strict)"(error in=w392, "Visible"=w391) -> (error out=w393:errorcluster)  [unwired: 1 in, 1 out]
                }
                frame 4 {
                  n221 = local read "MCS"() -> (w394:bool)
                  n222 = property on="MCS" class="Bool (strict)"(error in=w395, "Visible"=w394) -> (error out=w396:errorcluster)  [unwired: 1 in, 1 out]
                }
                frame 5 {
                  n223 = local read "LaserLocking"() -> (w397:bool)
                  n224 = property on="LaserLocking" class="Bool (strict)"(error in=w398, "Visible"=w397) -> (error out=w399:errorcluster)  [unwired: 1 in, 1 out]
                }
                frame 6 {
                  n225 = local read "Wavemeter"() -> (w400:bool)
                  n226 = property on="Wavemeter" class="Bool (strict)"(error in=w402, "Visible"=w400) -> (error out=w401:errorcluster)  [unwired: 1 in, 1 out]
                }
                frame 7 {
                  n227 = local read "Thermocouples"() -> (w403:bool)
                  n228 = property on="Thermocouples" class="Bool (strict)"(error in=w404, "Visible"=w403) -> (error out=w405:errorcluster)  [unwired: 1 in, 1 out]
                }
                frame 8 {
                  n229 = local read "Switches"() -> (w406:bool)
                  n230 = property on="Switches" class="Bool (strict)"(error in=w407, "Visible"=w406) -> (error out=w408:errorcluster)  [unwired: 1 in, 1 out]
                }
                frame 9 {
                  n231 = local read "QComposer"() -> (w409:bool)
                  n232 = property on="QComposer" class="Bool (strict)"(error in=w410, "Visible"=w409) -> (error out=w411:errorcluster)  [unwired: 1 in, 1 out]
                }
                frame 10 {
                  n233 = local read "UPS"() -> (w412:bool)
                  n234 = property on="UPS" class="Bool (strict)"(error in=w413, "Visible"=w412) -> (error out=w414:errorcluster)  [unwired: 1 in, 1 out]
                }
                frame 11 {
                  n235 = local read "PowerSwitches"() -> (w415:bool)
                  n236 = property on="PowerSwitches" class="Bool (strict)"(error in=w417, "Visible"=w415) -> (error out=w416:errorcluster)  [unwired: 1 in, 1 out]
                }
                frame 12 {
                  n237 = local read "Thor8000"() -> (w418:bool)
                  n238 = property on="Thor8000" class="Bool (strict)"(error in=w420, "Visible"=w418) -> (error out=w419:errorcluster)  [unwired: 1 in, 1 out]
                }
                frame 13 {
                  n239 = local read "Humidity"() -> (w421:bool)
                  n240 = property on="Humidity" class="Bool (strict)"(error in=w423, "Visible"=w421) -> (error out=w422:errorcluster)  [unwired: 1 in, 1 out]
                }
                frame 14 {
                  n241 = local read "TempScan"() -> (w424:bool)
                  n242 = property on="TempScan" class="Bool (strict)"(error in=w426, "Visible"=w424) -> (error out=w425:errorcluster)  [unwired: 1 in, 1 out]
                }
                frame 15 {
                  n243 = local read "NetCDF"() -> (w427:bool)
                  n244 = property on="NetCDF" class="Bool (strict)"(error in=w429, "Visible"=w427) -> (error out=w428:errorcluster)  [unwired: 1 in, 1 out]
                }
                frame 16 {
                  n245 = local read "Housekeeping"() -> (w430:bool)
                  n246 = property on="Housekeeping" class="Bool (strict)"(error in=w432, "Visible"=w430) -> (error out=w431:errorcluster)  [unwired: 1 in, 1 out]
                }
                frame 17 {
                  n247 = local read "ConfigQC"() -> (w435:bool)
                  n248 = property on="ConfigQC" class="Bool (strict)"(error in=w433, "Visible"=w435) -> (error out=w434:errorcluster)  [unwired: 1 in, 1 out]
                }
                frame 18 {
                  n249 = local read "SetupRScan"() -> (w438:bool)
                  n250 = property on="SetupRScan" class="Bool (strict)"(error in=w437, "Visible"=w438) -> (error out=w436:errorcluster)  [unwired: 1 in, 1 out]
                }
                frame 19 {
                  n251 = local read "ConfigThor8000"() -> (w441:bool)
                  n252 = property on="ConfigThor8000" class="Bool (strict)"(error in=w440, "Visible"=w441) -> (error out=w439:errorcluster)  [unwired: 1 in, 1 out]
                }
                frame 20 {
                  n253 = local read "CurrentSensor"() -> (w444:bool)
                  n254 = property on="CurrentSensor" class="Bool (strict)"(error in=w443, "Visible"=w444) -> (error out=w442:errorcluster)  [unwired: 1 in, 1 out]
                }
                frame 21 {
                  n255 = local read "TCSPC"() -> (w447:bool)
                  n256 = property on="TCSPC" class="Bool (strict)"(error in=w446, "Visible"=w447) -> (error out=w445:errorcluster)  [unwired: 1 in, 1 out]
                }
                frame 22 {
                  n257 = local read "Aerodiode"() -> (w449:bool)
                  n258 = property on="Aerodiode" class="Bool (strict)"(error in=w448, "Visible"=w449) -> (error out=w450:errorcluster)  [unwired: 1 in, 1 out]
                }
                frame 23 {
                  n259 = local read "BDetector"() -> (w453:bool)
                  n260 = property on="BDetector" class="Bool (strict)"(error in=w451, "Visible"=w453) -> (error out=w452:errorcluster)  [unwired: 1 in, 1 out]
                }
                frame 24 {
                  n261 = local read "DopFreeScan"() -> (w454:bool)
                  n262 = property on="DopFreeScan" class="Bool (strict)"(error in=w455, "Visible"=w454) -> (error out=w456:errorcluster)  [unwired: 1 in, 1 out]
                }
              }
            }
            n263 = Not(x=w373) -> (.not. x?=w374:bool)
            n264 = local write "First/LastCall"(w374) -> ()
          }
        }
      }
      frame "Idle" {
        n265 = while {
          tunnel: w463 -> [w546]
          shift-right: [w541] -> w464
          shift-left: w458 -> [w542]
          tunnel: [w540] -> w460
          tunnel: [w539] -> w457
          i -> [w543]
          stop <- w544 stop-if-true
          n266 = event shown="[24] \"PulsedScan\": Value Change" {
            selector: _ -> [_ _ _ _ _ _ _ _ _ _ _ _ _ _ _ _ _ _ _ _ _ _ _ _ _ _ _ _ _ _ _ _]
            dyn-events: _ -> [_ _ _ _ _ _ _ _ _ _ _ _ _ _ _ _ _ _ _ _ _ _ _ _ _ _ _ _ _ _ _ _]
            timeout: 100 -> [w558 _ _ _ _ _ _ _ _ _ _ _ _ _ _ _ _ _ _ _ _ _ _ _ _ _ _ _ _ _ _ _]
            tunnel: w546 -> [w553 w573 w580 w585 w589 w602 w614 w633 w645 w665 w684 w695 w706 w717 w728 w739 w750 w761 w772 w783 w794 w806 w824 w840 w855 w870 w881 w892 w903 w913 w925 w936]
            tunnel: [_ "Global Abort" TRUE ("Global Abort") _ _ TRUE ("Global Abort") TRUE ("Global Abort") TRUE ("Global Abort") TRUE ("Global Abort") TRUE ("Global Abort") TRUE ("Global Abort") TRUE ("Global Abort") TRUE ("Global Abort") TRUE ("Global Abort") TRUE ("Global Abort") TRUE ("Global Abort") TRUE ("Global Abort") TRUE ("Global Abort") TRUE ("Global Abort") TRUE ("Global Abort") TRUE ("Global Abort") TRUE ("Global Abort") TRUE ("Global Abort") TRUE ("Global Abort") TRUE ("Global Abort") TRUE ("Global Abort") TRUE ("Global Abort") TRUE ("Global Abort") TRUE ("Global Abort") TRUE ("Global Abort") TRUE ("Global Abort") TRUE ("Global Abort")] -> w544
            tunnel: w543 -> [w559 _ _ _ _ _ _ _ _ _ _ _ _ _ _ _ _ _ _ _ _ _ _ _ _ _ _ _ _ _ _ _]
            tunnel: w542 -> [w555 w576 w583 w588 w592 w604 w616 w635 w647 w667 w686 w697 w708 w719 w730 w741 w752 w763 w774 w785 w796 w808 w826 w842 w857 w872 w883 w894 w905 w915 w927 w938]
            tunnel: [w554 w575 w582 w587 w591 w603 w615 w634 w646 w666 w685 w696 w707 w718 w729 w740 w751 w762 w773 w784 w795 w807 w825 w841 w856 w871 w882 w893 w904 w914 w926 w937] -> w541
            tunnel: [w562 w572 w579 w584 w590 w594 w609 w626 w640 w660 w677 w688 w698 w709 w720 w732 w742 w753 w764 w776 w786 w801 w817 w833 w848 w863 w873 w884 w895 w906 w917 w928] -> w540
            tunnel: [_ _ _ _ _ w598 w610 w629 w641 w661 w680 w691 w702 w713 w724 w735 w746 w757 w768 w779 w790 w802 w827 w836 w851 w866 w877 w888 w899 w916 w921 w932] -> w539
            event Timeout {
              n267 = event-data() -> ()  [unwired: 1 in, 1 out]
              n268 = local read "AfterPulse Calibration"() -> (w551:bool)
              n269 = local read "Doppler Free Calibration"() -> (w550:bool)
              n270 = local read "Receiver Calibration"() -> (w552:bool)
              n271 = call "Idle_CollectionFreqCalc.vi"("Update Period (sec)"=10.0, "Individual Loop Wait Time(ms)"=w558, "Loop Itteration"=w559) -> ("Data Collect This Itteration?"=w556:bool)  [unwired: 8 in]
              n272 = local read "Children Responding"() -> (w565:T3)
              n273 = local read "ChildrenDetails"() -> (w548:T2)
              n274 = Build Array(w551, w550, w552) -> (w549:bool[])
              n275 = Boolean Array To Number(Boolean array=w549) -> (number=w547:u32)
              n276 = call "Idle_MainIdleProcess.vi"("ChildrenResponding"=w565, "QueueIn"=w555, "WriteStatus"=w556, "ChildrenDetailsIn"=w548, "CalibrationState"=w547, "ErrorIn"=w553) -> ("QueueOut"=w554:refnum<queue>, "ChildrenResponding"=→"Children Responding":T3, "ErrorOut"=w561:errorcluster, "ComandedStop"=w563:bool, "ChildrenDetailsOut"=w566:T10[])  [unwired: 5 in]
              n277 = global write "WVDIAL_GlobalVariables.vi" "Children Details"(w566) -> ()
              n278 = case shown="True" w563 {
                tunnel: w561 -> [w568 w571]
                tunnel: [w568 w570] -> w562
                frame False {
                }
                frame True {
                  n279 = property on="UPSAbort" class="Bool (strict)"(error in=w571, "Val(Sgnl)"=TRUE ("Value (Signaling)")) -> (error out=w570:errorcluster)  [unwired: 1 in, 1 out]
                }
              }
              n280 = global read "WVDIAL_GlobalVariables.vi" "Configuration"() -> (→"Configuration":T13)
              n281 = global read "WVDIAL_GlobalVariables.vi" "PermissionLevel"() -> (→"Permission Level":i32)
              "LoopCounter" <- w559
            }
            event "Global Abort": Value Change {
              n282 = event-data() -> ()  [unwired: 1 in, 1 out]
              n283 = Enqueue Element At Opposite End(queue=w576, element="Exit", error in (no error)=w573) -> (queue out=w575:refnum<queue>, error out=w572:errorcluster)  [unwired: 1 in, 1 out]
              n284 = global write "WVDIAL_GlobalVariables.vi" "GlobalStop"("Global Abort") -> ()
            }
            event "UPSAbort": Value Change {
              n285 = event-data() -> ()  [unwired: 1 in, 1 out]
              n286 = Enqueue Element At Opposite End(queue=w583, element="Exit", error in (no error)=w580) -> (queue out=w582:refnum<queue>, error out=w579:errorcluster)  [unwired: 1 in, 1 out]
            }
            event "Update Permissions": Value Change {
              n287 = event-data() -> ()  [unwired: 1 in, 1 out]
              n288 = Enqueue Element(queue=w588, element="System_OpenPermissionsVI", error in (no error)=w585) -> (queue out=w587:refnum<queue>, error out=w584:errorcluster)  [unwired: 1 in, 1 out]
            }
            event "User Comment": Value Change {
              n289 = event-data() -> ()  [unwired: 1 in, 1 out]
              n290 = Enqueue Element(queue=w592, element="System_OpenUserCommentVI", error in (no error)=w589) -> (queue out=w591:refnum<queue>, error out=w590:errorcluster)  [unwired: 1 in, 1 out]
            }
            event "Software Testing": Value Change {
              n291 = event-data() -> ()  [unwired: 1 in, 1 out]
              n292 = Enqueue Element At Opposite End(queue=w604, element="Exit", error in (no error)=w602) -> (queue out=w603:refnum<queue>, error out=w600:errorcluster)  [unwired: 1 in, 1 out]
              n293 = call "Idle_CommandChildrenExit.vi"("ErrorIn"=w600) -> ("ErrorOut"=w594:errorcluster)  [unwired: 4 in]
              n294 = Select(t=TypeDef_ConfigureFIleTypes."Main" ("MainControlSystems"), s=TRUE, f=TypeDef_ConfigureFIleTypes."Main" ("MainControlSystems")) -> (s? t:f=w598:T7)
            }
            event "Aerodiode": Value Change {
              n295 = event-data() -> ()  [unwired: 1 in, 1 out]
              n296 = Enqueue Element At Opposite End(queue=w616, element="Exit", error in (no error)=w614) -> (queue out=w615:refnum<queue>, error out=w612:errorcluster)  [unwired: 1 in, 1 out]
              n297 = call "Idle_CommandChildrenExit.vi"("ErrorIn"=w612) -> ("ErrorOut"=w609:errorcluster)  [unwired: 4 in]
              n298 = local read "Permission Level"() -> (w608:T4)
              n299 = Greater Or Equal?(x=w608, y=T4."Unset") -> (x >= y?=w606:bool)
              n300 = case shown="False" w606 {
                tunnel: [w620 w624] -> w610
                tunnel: "Aerodiode" -> [w617 w621]
                frame True {
                  n301 = Select(t=TypeDef_ConfigureFIleTypes."Main" ("MainControlSystems"), s=w617, f=TypeDef_ConfigureFIleTypes."ConfigureAerodiode" ("MainControlSystems")) -> (s? t:f=w620:T7)
                }
                frame False {
                  n302 = Select(t=TypeDef_ConfigureFIleTypes."Main" ("MainControlSystems"), s=w621, f=TypeDef_ConfigureFIleTypes."OpsTemplate" ("MainControlSystems")) -> (s? t:f=w624:T7)
                }
              }
            }
            event "BDetector": Value Change {
              n303 = event-data() -> ()  [unwired: 1 in, 1 out]
              n304 = Enqueue Element At Opposite End(queue=w635, element="Exit", error in (no error)=w633) -> (queue out=w634:refnum<queue>, error out=w631:errorcluster)  [unwired: 1 in, 1 out]
              n305 = call "Idle_CommandChildrenExit.vi"("ErrorIn"=w631) -> ("ErrorOut"=w626:errorcluster)  [unwired: 4 in]
              n306 = Select(t=TypeDef_ConfigureFIleTypes."Main" ("MainControlSystems"), s="BDetector", f=TypeDef_ConfigureFIleTypes."TestingBalancedDetector" ("MainControlSystems")) -> (s? t:f=w629:T7)
            }
            event "ConfigQC": Value Change {
              n307 = event-data() -> ()  [unwired: 1 in, 1 out]
              n308 = Enqueue Element At Opposite End(queue=w647, element="Exit", error in (no error)=w645) -> (queue out=w646:refnum<queue>, error out=w643:errorcluster)  [unwired: 1 in, 1 out]
              n309 = call "Idle_CommandChildrenExit.vi"("ErrorIn"=w643) -> ("ErrorOut"=w640:errorcluster)  [unwired: 4 in]
              n310 = local read "Permission Level"() -> (w638:T4)
              n311 = Greater Or Equal?(x=w638, y=T4."Administrator") -> (x >= y?=w636:bool)
              n312 = case shown="False" w636 {
                tunnel: [w651 w655] -> w641
                tunnel: "ConfigQC" -> [w648 w652]
                frame True {
                  n313 = Select(t=TypeDef_ConfigureFIleTypes."Main" ("MainControlSystems"), s=w648, f=TypeDef_ConfigureFIleTypes."ConfigureQC" ("MainControlSystems")) -> (s? t:f=w651:T7)
                }
                frame False {
                  n314 = Select(t=TypeDef_ConfigureFIleTypes."Main" ("MainControlSystems"), s=w652, f=TypeDef_ConfigureFIleTypes."OpsTemplate" ("MainControlSystems")) -> (s? t:f=w655:T7)
                }
              }
            }
            event "ConfigThor8000": Value Change {
              n315 = event-data() -> ()  [unwired: 1 in, 1 out]
              n316 = Enqueue Element At Opposite End(queue=w667, element="Exit", error in (no error)=w665) -> (queue out=w666:refnum<queue>, error out=w663:errorcluster)  [unwired: 1 in, 1 out]
              n317 = call "Idle_CommandChildrenExit.vi"("ErrorIn"=w663) -> ("ErrorOut"=w660:errorcluster)  [unwired: 4 in]
              n318 = local read "Permission Level"() -> (w657:T4)
              n319 = Greater Or Equal?(x=w657, y=T4."Administrator") -> (x >= y?=w656:bool)
              n320 = case shown="True" w656 {
                tunnel: [w671 w675] -> w661
                tunnel: "ConfigThor8000" -> [w668 w672]
                frame True {
                  n321 = Select(t=TypeDef_ConfigureFIleTypes."Main" ("MainControlSystems"), s=w668, f=TypeDef_ConfigureFIleTypes."ConfigureThor8000" ("MainControlSystems")) -> (s? t:f=w671:T7)
                }
                frame False {
                  n322 = Select(t=TypeDef_ConfigureFIleTypes."Main" ("MainControlSystems"), s=w672, f=TypeDef_ConfigureFIleTypes."OpsTemplate" ("MainControlSystems")) -> (s? t:f=w675:T7)
                }
              }
            }
            event "CurrentSensor": Value Change {
              n323 = event-data() -> ()  [unwired: 1 in, 1 out]
              n324 = Enqueue Element At Opposite End(queue=w686, element="Exit", error in (no error)=w684) -> (queue out=w685:refnum<queue>, error out=w682:errorcluster)  [unwired: 1 in, 1 out]
              n325 = call "Idle_CommandChildrenExit.vi"("ErrorIn"=w682) -> ("ErrorOut"=w677:errorcluster)  [unwired: 4 in]
              n326 = Select(t=TypeDef_ConfigureFIleTypes."Main" ("MainControlSystems"), s="CurrentSensor", f=TypeDef_ConfigureFIleTypes."OpsCurrent" ("MainControlSystems")) -> (s? t:f=w680:T7)
            }
            event "Housekeeping": Value Change {
              n327 = event-data() -> ()  [unwired: 1 in, 1 out]
              n328 = Enqueue Element At Opposite End(queue=w697, element="Exit", error in (no error)=w695) -> (queue out=w696:refnum<queue>, error out=w693:errorcluster)  [unwired: 1 in, 1 out]
              n329 = call "Idle_CommandChildrenExit.vi"("ErrorIn"=w693) -> ("ErrorOut"=w688:errorcluster)  [unwired: 4 in]
              n330 = Select(t=TypeDef_ConfigureFIleTypes."Main" ("MainControlSystems"), s="Housekeeping", f=TypeDef_ConfigureFIleTypes."OpsHousekeeping" ("MainControlSystems")) -> (s? t:f=w691:T7)
            }
            event "Humidity": Value Change {
              n331 = event-data() -> ()  [unwired: 1 in, 1 out]
              n332 = Enqueue Element At Opposite End(queue=w708, element="Exit", error in (no error)=w706) -> (queue out=w707:refnum<queue>, error out=w704:errorcluster)  [unwired: 1 in, 1 out]
              n333 = call "Idle_CommandChildrenExit.vi"("ErrorIn"=w704) -> ("ErrorOut"=w698:errorcluster)  [unwired: 4 in]
              n334 = Select(t=TypeDef_ConfigureFIleTypes."Main" ("MainControlSystems"), s="Humidity", f=TypeDef_ConfigureFIleTypes."OpsHumiditySensor" ("MainControlSystems")) -> (s? t:f=w702:T7)
            }
            event "LaserLocking": Value Change {
              n335 = event-data() -> ()  [unwired: 1 in, 1 out]
              n336 = Enqueue Element At Opposite End(queue=w719, element="Exit", error in (no error)=w717) -> (queue out=w718:refnum<queue>, error out=w715:errorcluster)  [unwired: 1 in, 1 out]
              n337 = call "Idle_CommandChildrenExit.vi"("ErrorIn"=w715) -> ("ErrorOut"=w709:errorcluster)  [unwired: 4 in]
              n338 = Select(t=TypeDef_ConfigureFIleTypes."Main" ("MainControlSystems"), s="LaserLocking", f=TypeDef_ConfigureFIleTypes."OpsWavlengthLocking" ("MainControlSystems")) -> (s? t:f=w713:T7)
            }
            event "MCS": Value Change {
              n339 = event-data() -> ()  [unwired: 1 in, 1 out]
              n340 = Enqueue Element At Opposite End(queue=w730, element="Exit", error in (no error)=w728) -> (queue out=w729:refnum<queue>, error out=w726:errorcluster)  [unwired: 1 in, 1 out]
              n341 = call "Idle_CommandChildrenExit.vi"("ErrorIn"=w726) -> ("ErrorOut"=w720:errorcluster)  [unwired: 4 in]
              n342 = Select(t=TypeDef_ConfigureFIleTypes."Main" ("MainControlSystems"), s="MCS", f=TypeDef_ConfigureFIleTypes."OpsMCS" ("MainControlSystems")) -> (s? t:f=w724:T7)
            }
            event "NetCDF": Value Change {
              n343 = event-data() -> ()  [unwired: 1 in, 1 out]
              n344 = Enqueue Element At Opposite End(queue=w741, element="Exit", error in (no error)=w739) -> (queue out=w740:refnum<queue>, error out=w737:errorcluster)  [unwired: 1 in, 1 out]
              n345 = call "Idle_CommandChildrenExit.vi"("ErrorIn"=w737) -> ("ErrorOut"=w732:errorcluster)  [unwired: 4 in]
              n346 = Select(t=TypeDef_ConfigureFIleTypes."Main" ("MainControlSystems"), s="NetCDF", f=TypeDef_ConfigureFIleTypes."OpsNetCDF" ("MainControlSystems")) -> (s? t:f=w735:T7)
            }
            event "Operations": Value Change {
              n347 = event-data() -> ()  [unwired: 1 in, 1 out]
              n348 = Enqueue Element At Opposite End(queue=w752, element="Exit", error in (no error)=w750) -> (queue out=w751:refnum<queue>, error out=w748:errorcluster)  [unwired: 1 in, 1 out]
              n349 = call "Idle_CommandChildrenExit.vi"("ErrorIn"=w748) -> ("ErrorOut"=w742:errorcluster)  [unwired: 4 in]
              n350 = Select(t=TypeDef_ConfigureFIleTypes."Main" ("MainControlSystems"), s="Operations", f=TypeDef_ConfigureFIleTypes."OpsMain" ("MainControlSystems")) -> (s? t:f=w746:T7)
            }
            event "PowerSwitches": Value Change {
              n351 = event-data() -> ()  [unwired: 1 in, 1 out]
              n352 = Enqueue Element At Opposite End(queue=w763, element="Exit", error in (no error)=w761) -> (queue out=w762:refnum<queue>, error out=w759:errorcluster)  [unwired: 1 in, 1 out]
              n353 = call "Idle_CommandChildrenExit.vi"("ErrorIn"=w759) -> ("ErrorOut"=w753:errorcluster)  [unwired: 4 in]
              n354 = Select(t=TypeDef_ConfigureFIleTypes."Main" ("MainControlSystems"), s="PowerSwitches", f=TypeDef_ConfigureFIleTypes."TestingPowerSwitches" ("MainControlSystems")) -> (s? t:f=w757:T7)
            }
            event "QComposer": Value Change {
              n355 = event-data() -> ()  [unwired: 1 in, 1 out]
              n356 = Enqueue Element At Opposite End(queue=w774, element="Exit", error in (no error)=w772) -> (queue out=w773:refnum<queue>, error out=w770:errorcluster)  [unwired: 1 in, 1 out]
              n357 = call "Idle_CommandChildrenExit.vi"("ErrorIn"=w770) -> ("ErrorOut"=w764:errorcluster)  [unwired: 4 in]
              n358 = Select(t=TypeDef_ConfigureFIleTypes."Main" ("MainControlSystems"), s="QComposer", f=TypeDef_ConfigureFIleTypes."OpsQuantumComposer" ("MainControlSystems")) -> (s? t:f=w768:T7)
            }
            event "SetupRScan": Value Change {
              n359 = event-data() -> ()  [unwired: 1 in, 1 out]
              n360 = Enqueue Element At Opposite End(queue=w785, element="Exit", error in (no error)=w783) -> (queue out=w784:refnum<queue>, error out=w781:errorcluster)  [unwired: 1 in, 1 out]
              n361 = call "Idle_CommandChildrenExit.vi"("ErrorIn"=w781) -> ("ErrorOut"=w776:errorcluster)  [unwired: 4 in]
              n362 = Select(t=TypeDef_ConfigureFIleTypes."Main" ("MainControlSystems"), s="SetupRScan", f=TypeDef_ConfigureFIleTypes."TestingSetupReceiverScan" ("MainControlSystems")) -> (s? t:f=w779:T7)
            }
            event "Switches": Value Change {
              n363 = event-data() -> ()  [unwired: 1 in, 1 out]
              n364 = Enqueue Element At Opposite End(queue=w796, element="Exit", error in (no error)=w794) -> (queue out=w795:refnum<queue>, error out=w792:errorcluster)  [unwired: 1 in, 1 out]
              n365 = call "Idle_CommandChildrenExit.vi"("ErrorIn"=w792) -> ("ErrorOut"=w786:errorcluster)  [unwired: 4 in]
              n366 = Select(t=TypeDef_ConfigureFIleTypes."Main" ("MainControlSystems"), s="Switches", f=TypeDef_ConfigureFIleTypes."TestingSwitches" ("MainControlSystems")) -> (s? t:f=w790:T7)
            }
            event "TCSPC": Value Change {
              n367 = event-data() -> ()  [unwired: 1 in, 1 out]
              n368 = Enqueue Element At Opposite End(queue=w808, element="Exit", error in (no error)=w806) -> (queue out=w807:refnum<queue>, error out=w804:errorcluster)  [unwired: 1 in, 1 out]
              n369 = call "Idle_CommandChildrenExit.vi"("ErrorIn"=w804) -> ("ErrorOut"=w801:errorcluster)  [unwired: 4 in]
              n370 = local read "Permission Level"() -> (w799:T4)
              n371 = Greater Or Equal?(x=w799, y=T4."Administrator") -> (x >= y?=w798:bool)
              n372 = case shown="True" w798 {
                tunnel: [w812 w816] -> w802
                tunnel: "TCSPC" -> [w809 w813]
                frame True {
                  n373 = Select(t=TypeDef_ConfigureFIleTypes."Main" ("MainControlSystems"), s=w809, f=TypeDef_ConfigureFIleTypes."OpsTemplate" ("MainControlSystems")) -> (s? t:f=w812:T7)
                }
                frame False {
                  n374 = Select(t=TypeDef_ConfigureFIleTypes."Main" ("MainControlSystems"), s=w813, f=TypeDef_ConfigureFIleTypes."OpsTemplate" ("MainControlSystems")) -> (s? t:f=w816:T7)
                }
              }
            }
            event "Template": Value Change {
              n375 = event-data() -> ()  [unwired: 1 in, 1 out]
              n376 = Enqueue Element At Opposite End(queue=w826, element="Exit", error in (no error)=w824) -> (queue out=w825:refnum<queue>, error out=w819:errorcluster)  [unwired: 1 in, 1 out]
              n377 = call "Idle_CommandChildrenExit.vi"("ErrorIn"=w819) -> ("ErrorOut"=w817:errorcluster)  [unwired: 4 in]
              n378 = Select(t=TypeDef_ConfigureFIleTypes."Main" ("MainControlSystems"), s="Template", f=TypeDef_ConfigureFIleTypes."OpsTemplate" ("MainControlSystems")) -> (s? t:f=w827:T7)
            }
            event "TempScan": Value Change {
              n379 = event-data() -> ()  [unwired: 1 in, 1 out]
              n380 = Enqueue Element At Opposite End(queue=w842, element="Exit", error in (no error)=w840) -> (queue out=w841:refnum<queue>, error out=w838:errorcluster)  [unwired: 1 in, 1 out]
              n381 = call "Idle_CommandChildrenExit.vi"("ErrorIn"=w838) -> ("ErrorOut"=w833:errorcluster)  [unwired: 4 in]
              n382 = Select(t=TypeDef_MainSpecialConfiguration."Ops" ("Configuration"), s="TempScan", f=TypeDef_MainSpecialConfiguration."ReceiverScan" ("Configuration")) -> (s? t:f=w832:T13)
              n383 = global write "WVDIAL_GlobalVariables.vi" "Configuration"(w832) -> ()
              n384 = Not(x="TempScan") -> (.not. x?=→"Receiver Calibration":bool)
              n385 = Select(t=TypeDef_ConfigureFIleTypes."Main" ("MainControlSystems"), s="TempScan", f=TypeDef_ConfigureFIleTypes."TestingReceiverScan" ("MainControlSystems")) -> (s? t:f=w836:T7)
            }
            event "PulsedScan": Value Change {
              n386 = event-data() -> ()  [unwired: 1 in, 1 out]
              n387 = Enqueue Element At Opposite End(queue=w857, element="Exit", error in (no error)=w855) -> (queue out=w856:refnum<queue>, error out=w853:errorcluster)  [unwired: 1 in, 1 out]
              n388 = call "Idle_CommandChildrenExit.vi"("ErrorIn"=w853) -> ("ErrorOut"=w848:errorcluster)  [unwired: 4 in]
              n389 = Select(t=TypeDef_MainSpecialConfiguration."Ops" ("Configuration"), s="PulsedScan", f=TypeDef_MainSpecialConfiguration."PulsedScan" ("Configuration")) -> (s? t:f=w847:T13)
              n390 = Not(x="PulsedScan") -> (.not. x?=w844:bool)
              n391 = local write "Receiver Calibration"(w844) -> ()
              n392 = global write "WVDIAL_GlobalVariables.vi" "Configuration"(w847) -> ()
              n393 = Select(t=TypeDef_ConfigureFIleTypes."Main" ("MainControlSystems"), s="PulsedScan", f=TypeDef_ConfigureFIleTypes."TestingReceiverScan" ("MainControlSystems")) -> (s? t:f=w851:T7)
            }
            event "DopFreeScan": Value Change {
              n394 = event-data() -> ()  [unwired: 1 in, 1 out]
              n395 = Enqueue Element At Opposite End(queue=w872, element="Exit", error in (no error)=w870) -> (queue out=w871:refnum<queue>, error out=w868:errorcluster)  [unwired: 1 in, 1 out]
              n396 = call "Idle_CommandChildrenExit.vi"("ErrorIn"=w868) -> ("ErrorOut"=w863:errorcluster)  [unwired: 4 in]
              n397 = Select(t=TypeDef_MainSpecialConfiguration."Ops" ("Configuration"), s="DopFreeScan", f=TypeDef_MainSpecialConfiguration."HyperFineScan" ("Configuration")) -> (s? t:f=w862:T13)
              n398 = global write "WVDIAL_GlobalVariables.vi" "Configuration"(w862) -> ()
              n399 = Not(x="DopFreeScan") -> (.not. x?=→"Doppler Free Calibration":bool)
              n400 = Select(t=TypeDef_ConfigureFIleTypes."Main" ("MainControlSystems"), s="DopFreeScan", f=TypeDef_ConfigureFIleTypes."TestingHyperFineScan" ("MainControlSystems")) -> (s? t:f=w866:T7)
            }
            event "Thermocouples": Value Change {
              n401 = event-data() -> ()  [unwired: 1 in, 1 out]
              n402 = Enqueue Element At Opposite End(queue=w883, element="Exit", error in (no error)=w881) -> (queue out=w882:refnum<queue>, error out=w879:errorcluster)  [unwired: 1 in, 1 out]
              n403 = call "Idle_CommandChildrenExit.vi"("ErrorIn"=w879) -> ("ErrorOut"=w873:errorcluster)  [unwired: 4 in]
              n404 = Select(t=TypeDef_ConfigureFIleTypes."Main" ("MainControlSystems"), s="Thermocouples", f=TypeDef_ConfigureFIleTypes."OpsThermocouple" ("MainControlSystems")) -> (s? t:f=w877:T7)
            }
            event "Thor8000": Value Change {
              n405 = event-data() -> ()  [unwired: 1 in, 1 out]
              n406 = Enqueue Element At Opposite End(queue=w894, element="Exit", error in (no error)=w892) -> (queue out=w893:refnum<queue>, error out=w890:errorcluster)  [unwired: 1 in, 1 out]
              n407 = call "Idle_CommandChildrenExit.vi"("ErrorIn"=w890) -> ("ErrorOut"=w884:errorcluster)  [unwired: 4 in]
              n408 = Select(t=TypeDef_ConfigureFIleTypes."Main" ("MainControlSystems"), s="Thor8000", f=TypeDef_ConfigureFIleTypes."TestingThor8000" ("MainControlSystems")) -> (s? t:f=w888:T7)
            }
            event "UPS": Value Change {
              n409 = event-data() -> ()  [unwired: 1 in, 1 out]
              n410 = Enqueue Element At Opposite End(queue=w905, element="Exit", error in (no error)=w903) -> (queue out=w904:refnum<queue>, error out=w901:errorcluster)  [unwired: 1 in, 1 out]
              n411 = call "Idle_CommandChildrenExit.vi"("ErrorIn"=w901) -> ("ErrorOut"=w895:errorcluster)  [unwired: 4 in]
              n412 = Select(t=TypeDef_ConfigureFIleTypes."Main" ("MainControlSystems"), s="UPS", f=TypeDef_ConfigureFIleTypes."OpsUPS" ("MainControlSystems")) -> (s? t:f=w899:T7)
            }
            event "Warmup": Value Change {
              n413 = event-data() -> ()  [unwired: 1 in, 1 out]
              n414 = Enqueue Element At Opposite End(queue=w915, element="Exit", error in (no error)=w913) -> (queue out=w914:refnum<queue>, error out=w909:errorcluster)  [unwired: 1 in, 1 out]
              n415 = call "Idle_CommandChildrenExit.vi"("ErrorIn"=w909) -> ("ErrorOut"=w906:errorcluster)  [unwired: 4 in]
              n416 = Select(t=TypeDef_ConfigureFIleTypes."Main" ("MainControlSystems"), s="Warmup", f=TypeDef_ConfigureFIleTypes."OpsWarmup" ("MainControlSystems")) -> (s? t:f=w916:T7)
            }
            event "Wavemeter": Value Change {
              n417 = event-data() -> ()  [unwired: 1 in, 1 out]
              n418 = Enqueue Element At Opposite End(queue=w927, element="Exit", error in (no error)=w925) -> (queue out=w926:refnum<queue>, error out=w923:errorcluster)  [unwired: 1 in, 1 out]
              n419 = call "Idle_CommandChildrenExit.vi"("ErrorIn"=w923) -> ("ErrorOut"=w917:errorcluster)  [unwired: 4 in]
              n420 = Select(t=TypeDef_ConfigureFIleTypes."Main" ("MainControlSystems"), s="Wavemeter", f=TypeDef_ConfigureFIleTypes."TestingWavemeter" ("MainControlSystems")) -> (s? t:f=w921:T7)
            }
            event "Weather Station": Value Change {
              n421 = event-data() -> ()  [unwired: 1 in, 1 out]
              n422 = Enqueue Element At Opposite End(queue=w938, element="Exit", error in (no error)=w936) -> (queue out=w937:refnum<queue>, error out=w934:errorcluster)  [unwired: 1 in, 1 out]
              n423 = call "Idle_CommandChildrenExit.vi"("ErrorIn"=w934) -> ("ErrorOut"=w928:errorcluster)  [unwired: 4 in]
              n424 = Select(t=TypeDef_ConfigureFIleTypes."Main" ("MainControlSystems"), s="Weather Station", f=TypeDef_ConfigureFIleTypes."OpsWeatherStation" ("MainControlSystems")) -> (s? t:f=w932:T7)
            }
          }
        }
        n425 = while {
          tunnel: w458 -> [w471]
          tunnel: [w470] -> w462
          shift-right: [w467] -> w461
          shift-left: w463 -> [w472]
          i -> [w469]
          stop <- w468 stop-if-true
          n426 = case shown="No Error" w472 {
            selector: w472 -> [w482 w538]
            tunnel: w471 -> [w481 _]
            tunnel: [w489 _] -> w468
            tunnel: [w488 _] -> w470
            tunnel: [w487 w538] -> w466
            tunnel: w469 -> [_ _]
            tunnel: [w486 TRUE ("GlobalStop")] -> w465
            frame No Error {
              n427 = Dequeue Element(queue=w481, error in (no error)=w482) -> (element=w483:string, error out=w485:errorcluster)  [unwired: 1 in, 2 out]
              n428 = call "Idle_ParseStringCommand.vi"("error in"=w485, "Input Command"=w483) -> ("error out"=w484:errorcluster, "Command"=w480:string, "Remaining String"=w479:string)  [unwired: 1 in]
              n429 = case shown="\"False\", Default" w480 {
                tunnel: [w496 _ _] -> w489
                tunnel: [w495 _ _] -> w488
                tunnel: [w494 w518 w536] -> w487
                tunnel: [w492 TRUE ("GlobalStop") TRUE ("GlobalStop")] -> w486
                tunnel: w483 -> [w490 w521 _]
                tunnel: w484 -> [w491 w522 w525]
                tunnel: w479 -> [_ _ w533]
                frame "False", Default {
                  n430 = Equal?(x=w490, y="Exit") -> (x = y?=w497:bool)
                  n431 = case shown="False" w497 {
                    tunnel: w491 -> [w504 w512]
                    tunnel: w490 -> [w501 _]
                    tunnel: [_ TRUE] -> w496
                    tunnel: [_ w513] -> w495
                    tunnel: [w503 w512] -> w494
                    tunnel: "Software Testing" -> [w500 _]
                    tunnel: [TRUE ("GlobalStop") w511] -> w492
                    frame False {
                      n432 = case shown="False" w500 {
                        tunnel: w504 -> [w506 w510]
                        tunnel: [w506 w509] -> w503
                        tunnel: w501 -> [_ w508]
                        tunnel: ["" w507] -> w502
                        frame True {
                        }
                        frame False {
                          n433 = call "Idle_InterpretCommandsAndResponses.vi"("ErrorIn"=w510, "Input Command"=w508) -> ("ErrorOut"=w509:errorcluster, "What to Do"=w507:string)  [unwired: 4 in, 4 out]
                        }
                      }
                      "What to Do" <- w502
                    }
                    frame True {
                      n434 = global read "WVDIAL_GlobalVariables.vi" "GlobalStop"() -> (w511:bool)
                      n435 = Select(t=TypeDef_LoopStagesMain."Exit" ("Enum"), s=w511, f=TypeDef_LoopStagesMain."ExitChildren" ("Enum")) -> (s? t:f=w513:T6)
                    }
                  }
                  "QueueElement" <- w490
                }
                frame "ChildReport" {
                  n436 = local read "ChildrenDetails"() -> (w520:T2)
                  n437 = call "Idle_ParseChildResponse.vi"("ErrorIn"=w522, "ChildResponse"=w521, "ChildrenDetailsIn"=w520) -> ("ErrorOut"=w518:errorcluster, "ChildrenDetailsOut"=→"ChildrenDetails":T2)  [unwired: 1 in]
                }
                frame "WriteContainerData" {
                  n438 = local read "WritePaths"() -> (w531:path[])
                  n439 = local read "DataBasePath"() -> (w529:string)
                  n440 = local read "FileBaseNames"() -> (w530:string[])
                  n441 = local read "FileUpdateTime"() -> (w528:dbl)
                  n442 = call "Idle_GetTimeStamp.vi"() -> ("Fractional Hours"=w527:dbl)  [unwired: 11 in]
                  n443 = call "Idle_UpdateFileNamesOnTheHour.vi"("ErrorIn"=w525, "CurrentTime"=w527, "WritePathsIn"=w531, "FileBaseNamesIn"=w530, "DataBasePathIn"=w529, "FileUpdateTimeIn"=w528) -> ("WritePathsOut"=w524:path[], "FileUpdateTimeOut"=w526:dbl, "ErrorOur"=w523:errorcluster)  [unwired: 2 in, 1 out]
                  n444 = local write "WritePaths"(w524) -> ()
                  n445 = local write "FileUpdateTime"(w526) -> ()
                  n446 = Index Array(array=w524, index=0) -> (element=w532:path)
                  n447 = call "Idle_Write1DDataText.vi"("ErrorIn"=w523, "Write FilePath"=w532, "Data2Write"=w533) -> ("ErrorOut"=w536:errorcluster)  [unwired: 2 in]
                }
              }
            }
            frame Error {
            }
          }
          n448 = case shown="False" w465 {
            tunnel: w466 -> [_ w478]
            tunnel: [w475 w478] -> w467
            frame False {
              n449 = call "Exit_ChildExitListen.vi"() -> ("ErrorOut"=w474:errorcluster, "TimedOut"=w473:bool)  [unwired: 10 in]
              n450 = case shown="True" w473 {
                tunnel: w474 -> [w476 w477]
                tunnel: [w476 w477] -> w475
                frame False {
                }
                frame True {
                }
              }
            }
            frame True {
            }
          }
        }
        n451 = Merge Errors(w460, w461) -> (w459:errorcluster)
      }
      frame "ExitChildren" {
        n452 = local read "SubPanelRefs"() -> (w941:refnum<vi>[])
        n453 = for {
          tunnel: w941 -> [w945] mode=indexing
          shift-right: [w948] -> w940
          shift-left: w939 -> [w947]
          # "Removing subVIs\nfrom subPanels"
          n454 = Not A Number/Path/Refnum?(number/path/refnum=w945) -> (NaN/Path/Refnum?=w946:bool)
          n455 = case shown="False" w946 {
            tunnel: w945 -> [w951 _]
            tunnel: [w950 w952] -> w948
            tunnel: w947 -> [w949 w952]
            frame False {
              n456 = invoke class="SubPnl" method="Remove VI"(reference=w951, error in=w949) -> (error out=w950:errorcluster)  [unwired: 1 in, 2 out]
            }
            frame True {
            }
          }
        }
      }
      frame "Error Handler" {
        n457 = case shown="Error" w953 {
          selector: w953 -> [w957 w959]
          tunnel: [w957 w960] -> w954
          frame No Error {
          }
          frame Error {
            w966 = "\r\n"
            n458 = call "Idle_GetTimeStamp.vi"() -> ("Fractional Hours"=w967:dbl)  [unwired: 11 in]
            n459 = Number To Fractional String(number=w967, precision (6)=i16 5 ("width (-)")) -> (F-format string=w965:string)  [unwired: 2 in]
            n460 = Unbundle(w959) -> ("source"=w958:string)  [unwired: 2 out]
            n461 = local read "WritePaths"() -> (w962:path[])
            n462 = Concatenate Strings(w965, w966, w958, w966, w966) -> (w964:string)
            n463 = Index Array(array=w962, index=1) -> (element=w963:path)
            n464 = call "Idle_Write1DDataText.vi"("ErrorIn"=w959, "Write FilePath"=w963, "Data2Write"=w964) -> ("ErrorOut"=w960:errorcluster)  [unwired: 2 in]
          }
        }
      }
      frame "Exit" {
        w978 = FALSE
        w979 = TRUE ("Visible")
        w984 = T4."Unset" ("Permission Level")
        w983 = FALSE ("RunAsChild")
        # "Setting front panel size"
        n465 = property on="UPSAbort" class="Bool (strict)"(error in=w981, "Visible"=w979) -> (error out=w980:errorcluster)  [unwired: 1 in, 1 out]
        n466 = property on="First/LastCall" class="Bool (strict)"(error in=w980, "Visible"=w979) -> (error out=w982:errorcluster)  [unwired: 1 in, 1 out]
        n467 = global write "WVDIAL_GlobalVariables.vi" "Configuration"(enum16{"Ops", "ReceiverScan"}."Ops" ("Configuration")) -> ()
        n468 = global write "WVDIAL_GlobalVariables.vi" "RunAsChild"(w983) -> ()
        n469 = global write "WVDIAL_GlobalVariables.vi" "ChildAbort"(w983) -> ()
        n470 = local write "Permission Level"(w984) -> ()
        n471 = global write "WVDIAL_GlobalVariables.vi" "PermissionLevel"(w984) -> ()
        n472 = local read "Pages"() -> (w985:refnum<vi>[])
        n473 = for {
          shift-right: [w992] -> w971
          shift-left: w982 -> [w996]
          tunnel: w985 -> [w995] mode=indexing
          n474 = property class="Page"(reference=w995, error in=w996, "PageVis"=TRUE ("Page Visible")) -> (reference out=w991:refnum<vi>, error out=w993:errorcluster)
          n475 = Close Reference(reference=w991, error in (no error)=w993) -> (error out=w992:errorcluster)
        }
        n476 = Current VI's Path() -> (path=w972:path)
        n477 = Open VI Reference(vi path=w972, error in (no error)=w971) -> (vi reference=w973:refnum<vi>, error out=w974:errorcluster)  [unwired: 4 in]
        n478 = property class="VI"(reference=w973, error in=w974, "Front Panel.WinBounds"=T9 {"Left"=10, "Top"=30, "Right"=1310, "Bottom"=720} ("Front Panel Window:Panel Bounds"), "Front Panel.Closeable"=w978, "Front Panel.Resizeable"=w978) -> (reference out=w975:refnum<vi>, error out=w976:errorcluster)
        n479 = Close Reference(reference=w975, error in (no error)=w976) -> (error out=w970:errorcluster)
        n480 = property on="Children Responding" class="Arr (strict)"(error in=w970, "Visible"=TRUE) -> (error out=w987:errorcluster)  [unwired: 1 in, 1 out]
      }
    }
  }
  n481 = Release Queue(queue=w8, error in (no error)=w7) -> (error out=→"error IO":errorcluster)  [unwired: 1 in, 2 out]
